vi "eyecat MAX v02_JS.vi"() -> ()   [LabVIEW 2014]
doc: "This VI is an upgrade from the WIN 1_v4 that implements the ageing subrutine"
uses:
  Buttons/String output.ctl
  <vilib>/Utility/miscctls.llb/LVRowAndColumnTypeDef.ctl
  Buttons/Numeric control.ctl
  Buttons/String input.ctl
  Buttons/Numeric indicator.ctl
  Controls Win/Control 3.ctl
  <vilib>/Platform/TimedLoop/XDataNode/nitl_modes.ctl
  <vilib>/Platform/TimedLoop/XDataNode/timing_clust.ctl
  <vilib>/Platform/TimedLoop/XDataNode/wakeup.ctl
  <vilib>/Utility/file.llb/Read From Spreadsheet File (DBL).vi
  <vilib>/Utility/file.llb/Write To Spreadsheet File (string).vi
  <vilib>/Utility/file.llb/Read From Spreadsheet File (string).vi
  <vilib>/regexp/Match Regular Expression.xnode
  <vilib>/Platform/TimedLoop/XDataNode/XDataNode.xnode
  <vilib>/Platform/TimedLoop/XDataNode/XDNodeRunTimeDep.lvlib
panel:
  out "SO Valve 2":dbl[][](array[numeric]) format="%0.3f"
  out "SO Valve 1":dbl[][](array[numeric]) format="%0.3f"
  out "File name":string
  out "Log?":bool
  out "Advanced Logging":bool
  out "output cluster":T2
  out "Connected":bool
  out "Air Bal Array":dbl[][](array[numeric]) format="%0.3f"
  out "HC Array Bal":dbl[][](array[numeric]) format="%0.3f"
  out "Air Array":dbl[][](array[numeric]) format="%0.3f"
  out "HC Array Cyc":dbl[][](array[numeric]) format="%0.3f"
  out "MKS 1":i16
  out "MKS 2":i16
  out "Furnace temp 2":dbl
  out "Full system?":bool
  out "Log interval (seconds)":T1
  in  "Flow rate Age":dbl
  in  "Inlet temp Age":dbl
  out "Stopped?":bool
  in  "Stop Cmd":T1
  out "Connected?":bool
  out "Error":dbl
  out "Iteration Duration":i64
  out "Finished Late? [i-1]":bool
  in  "stop TCP":bool
  in  "SO2 ppm":dbl
  out "Furnace temp 1":dbl
  out "stop 2":bool
  in  "Enum 1":i16=1
  in  "Acknowledge":bool
  out "Test number":u16
  out "Flag1":bool=TRUE
  out "EditPos Subc":T3
  out "Flag 2":bool=TRUE
  in  "Tab Control":T4(tab)
  out "Doors Unlocked":bool
  in  "Temperature Limit (°C)":T1=800.0 min=0.0 max=1200.0 step=1.0
  in  "Log Test Button":bool
  in  "File Name":T5="Test"
  in  "File Path":path=path "C:/DATA LOG"
  out "Fail":bool
  out "Pass":bool
  in  "Select Test Type":T6(radio)
  out "Standby":bool
  out "Doors Open":bool
  out "Extractor Fan On":bool
  out "Test In Progress":bool
  out "Cool Down":bool
  out "System Alarm":bool
  in  "Execute Leak Test Button":bool
  in  "Stop Test Button":bool
  in  "Start Test Button":bool
  in  "Advanced settings":bool
  in  "Inlet Temperature (°C)":T1=400.0 min=350.0 max=1000.0 step=1.0
  in  "Inlet LAMBDA Rich":T1=0.9 min=0.85 max=0.96 step=0.001
  in  "Inlet LAMBDA Lean":T1=1.2 min=1.02 max=3.0 step=0.001
  in  "Test Stop temperature (°C)":T1=300.0 min=100.0 max=1000.0 step=1.0
  in  "Test Start Temperature (°C)":T1=125.0 min=0.0 max=500.0 step=1.0
  in  "Furnace Ramp Rate (°C/min)":T1=15.0 min=1.0 max=50.0 step=0.1
  in  "NO:CO Ratio":T1=1.1 min=1.0 max=5.0 step=0.1
  in  "Inlet O2 (%)":T1=0.5 min=0.0 max=14.0 step=0.01
  in  "Inlet LAMBDA":T1=1.0 min=0.6 max=3.0 step=0.001
  out "Space Velocity (h-1)":T7
  out "Vol Flow @ STP (l/min)":T7
  in  "Test Flow Rate(g/s)":T1 min=0.0 max=100.0 step=0.01
  out "Sample Volume (litres)":T7
  in  "Number of Samples":T1=1.0 min=1.0 max=6.0 step=1.0
  in  "Sample Diameter (mm)":T1
  out "CO Theory (%)":T7 format="%#_3g"
  out "CO Theory (%)":T7 format="%#_3g"
  out "HC Theory (%)":T7
  in  "Sample Length (mm)":T1 min=0.0 step=0.5
  in  "NO ppm SW":dbl=500.0 caption="NO (ppm)" min=0.0 max=500.0 step=1.0
  in  "NO ppm Loff":T1 caption="NO ppm"
  in  "Delete sCycle":bool
  in  "Load sCycle":bool
  in  "Save sCycle":bool
  in  "Clear subcycle":bool
  in  "Clear Cycle Pattern":bool
  in  "Save Cycle":bool
  in  "Load Cycle":bool
  in  "Delete Cycle":bool
  out "Test Compiled":bool
  in  "Compile Test Button":bool
  in  "Sub-Cycle List":i32(listbox)=1
  in  "Cycle List":i32(listbox)=2
  out "Total Test Duration (hrs)":T8
  in  "Ageing Gas":enum32{"Radio Selection 1", "Radio Selection 2"}(radio)
  in  "Sub-Cycle Pattern":string[][](table) caption="Subcycle pattern"
  in  "Total Number of Cycles":T1=1.0 min=1.0 max=10000.0 step=1.0
  in  "Cycle Pattern":string[][](table)
  in  "Sub-Cycle Name":T5
  in  "Cycle Name":T5
  out "Heat Exchanger Temperatures (°C)":dynamicdata(graph)
  out "Flow Rate (g/s)":dynamicdata(graph)
  out "Sample Temperatures (°C)":dynamicdata(graph)
  out "System Temperatures (°C)":dynamicdata(graph)
  out "HC Concentration (ppm)":dynamicdata(graph)
  out "Lambda":dynamicdata(graph)
  out "M584L Upstream & Downstream":dynamicdata(graph)
  out "NO Concentration (ppm)":dynamicdata(graph)
  in  "Purge System":bool
  in  "Alarm ack":bool
  in  "Clear log":bool
  out "Table":string[][](table)
  out "Soft Alarm":bool
  out "Hard Alarm":bool
  # "Test Type"
  # "Test Commands"
  # "System Indicators"
  # "Leak Test"
  # "Catalyst Specification"
  # "Lightoff Settings"
  # "Furnace Lightoff Settings"
  # "Sweep Settings"
  # "CO/HC Lightoff Settings"
  # "0.96 < lambda < 0.85"
  # "1.02< lambda < 1.6"
  # "350 < Tinlet < 1000"
  # "NO Lightoff Settings"
  # "Flow Specification"
  # "Cycle Compiled"
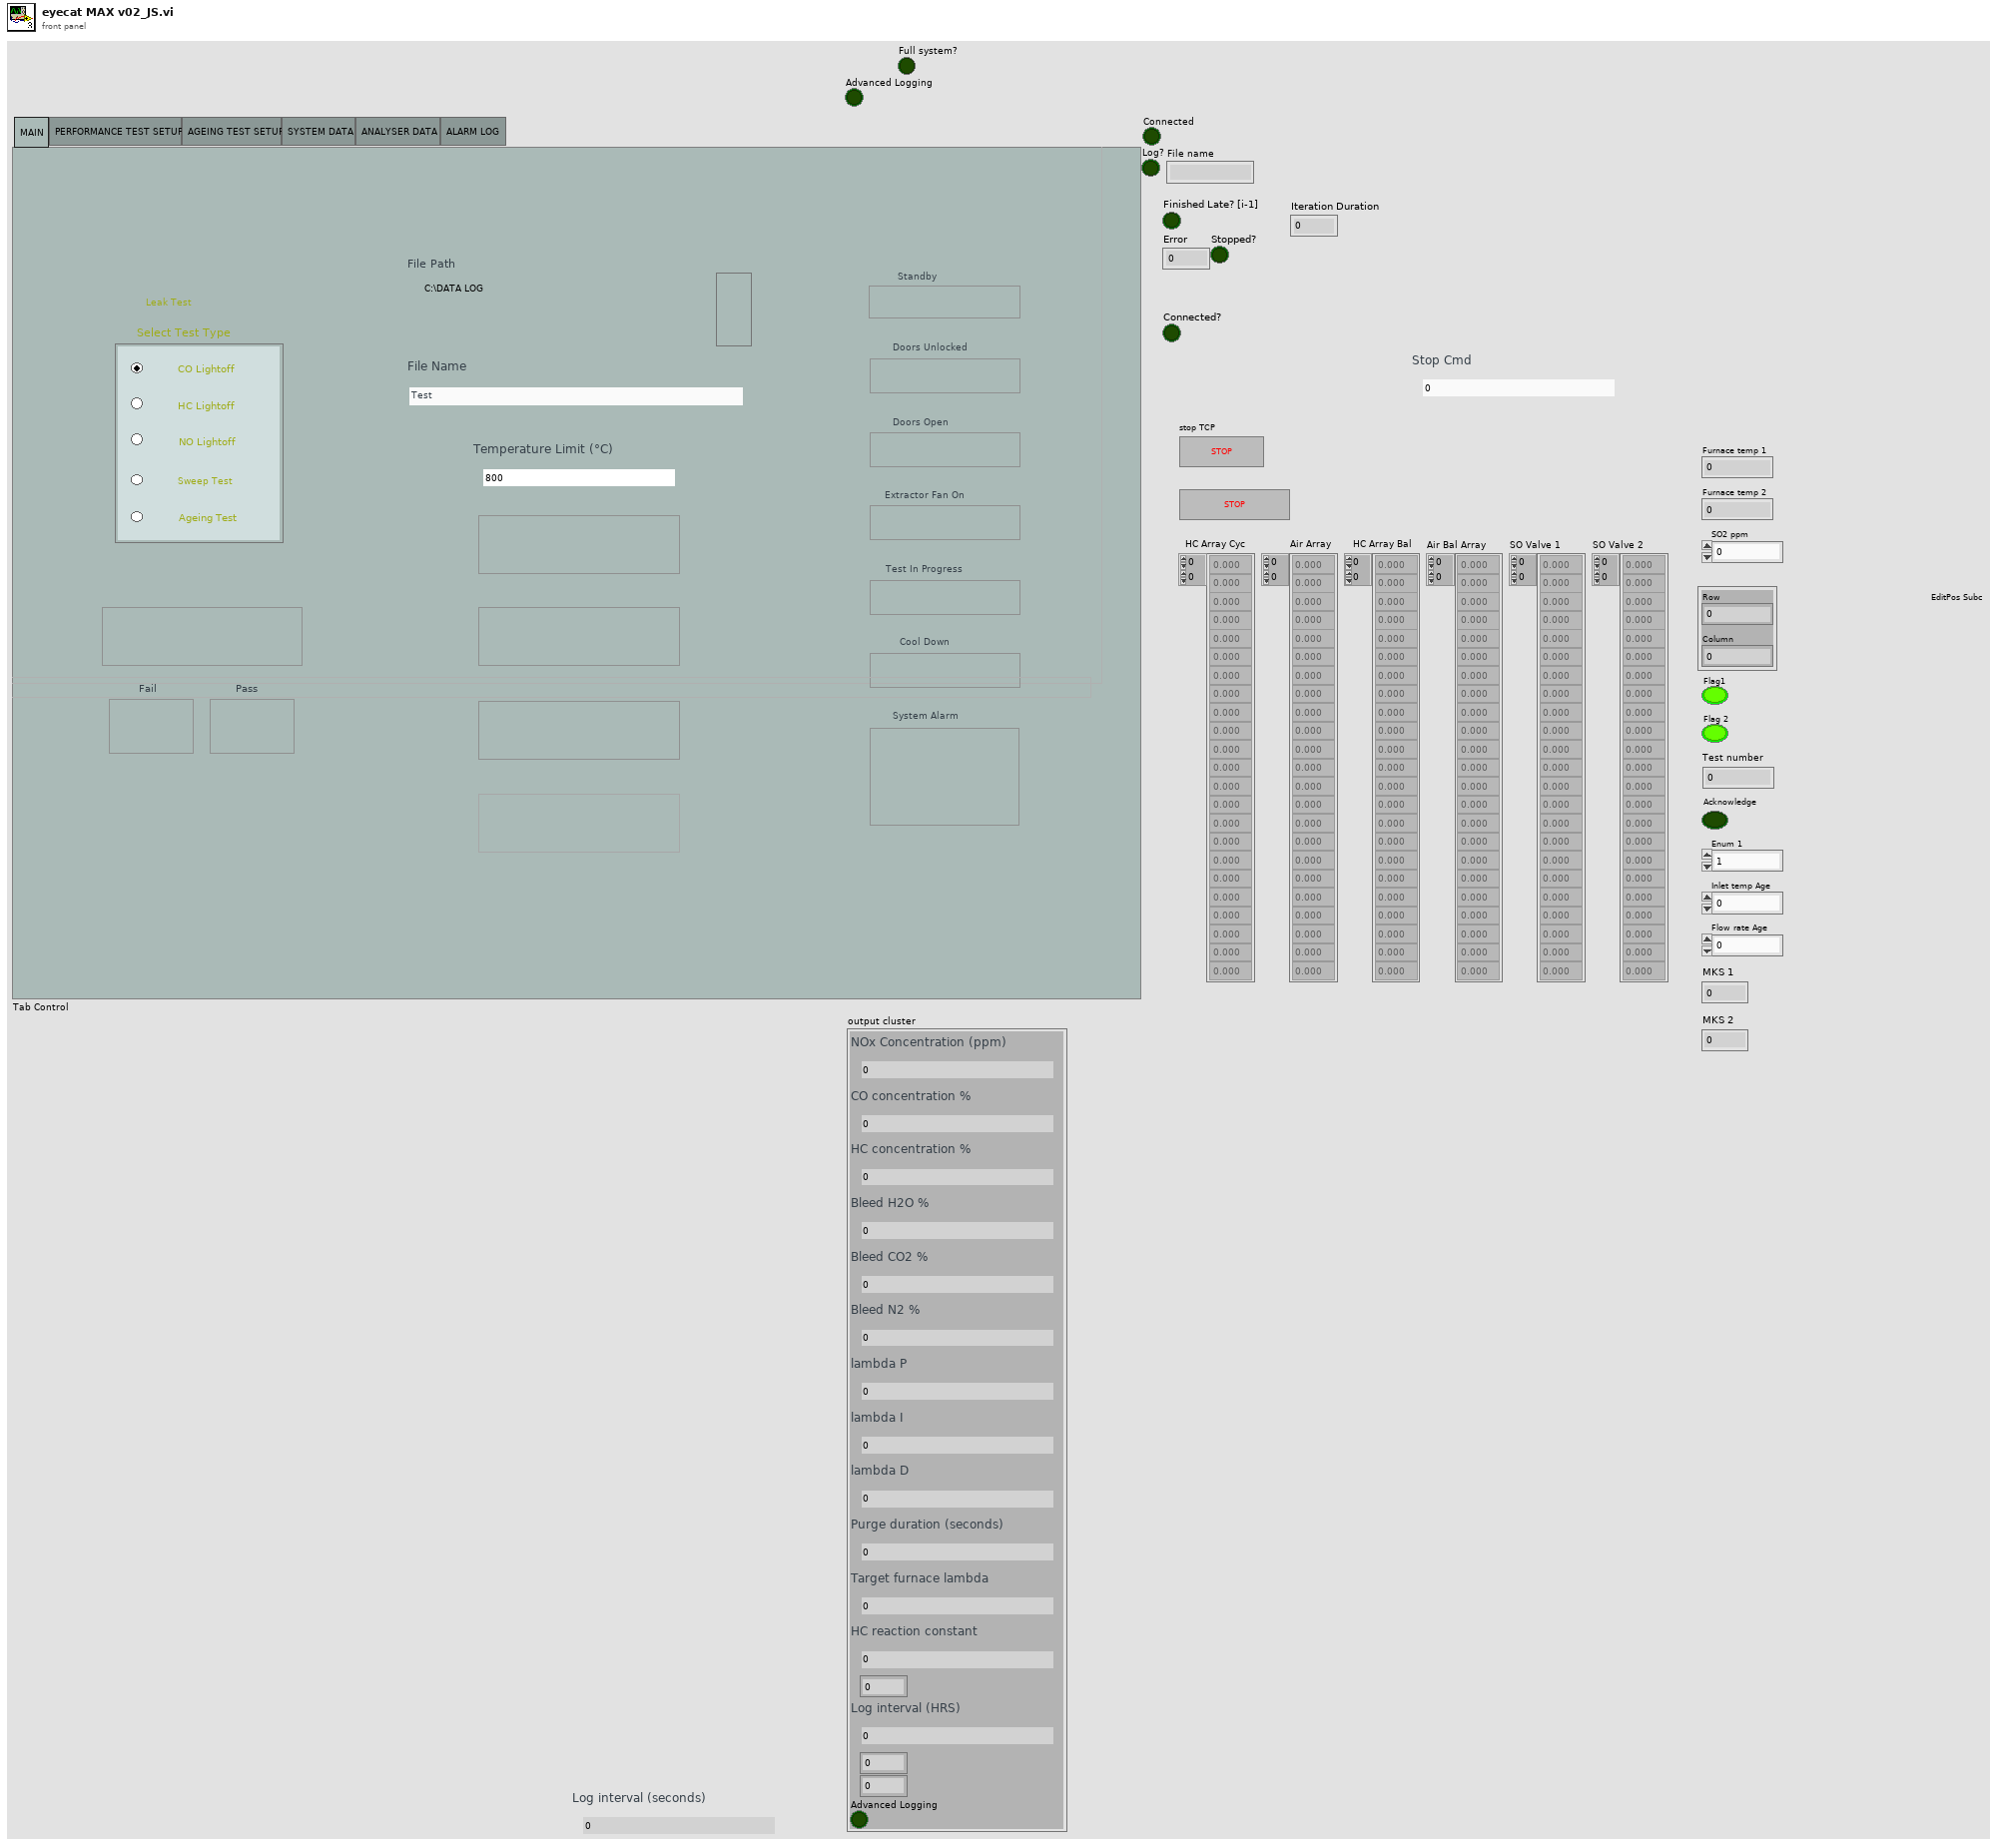
[diagram p1: front panel]
types:
  T1 = typedef "Numeric control.ctl" = dbl
  T2 = cluster{"NOx Concentration (ppm)":T1, "CO concentration %":T1, "HC concentration %":T1, "Bleed H2O %":T1, "Bleed CO2 %":T1, "Bleed N2 %":T1, "lambda P":T1, "lambda I":T1, "lambda D":T1, "Purge duration (seconds)":T1, "Target furnace lambda":T1, "HC reaction constant":T1, i16, "Log interval (HRS)":T1, i16, i16, "Advanced Logging":bool}
  T3 = typedef "LVRowAndColumnTypeDef.ctl" = cluster{"Row":i32, "Column":i32}
  T4 = enum32{"MAIN", "PERFORMANCE TEST SETUP", "AGEING TEST SETUP", "SYSTEM DATA", "ANALYSER DATA", "ALARM LOG"}
  T5 = typedef "String input.ctl" = string
  T6 = enum32{"CO Lightoff", "HC Lightoff", "NO Lightoff", "Sweep Test", "Ageing Test"}
  T7 = typedef "Numeric indicator.ctl" = dbl
  T8 = typedef "String output.ctl" = string
  T9 = typedef "XDNodeRunTimeDep.lvlib/nitl_modes.ctl" = enum32{"No Change", "Process missed periods, maintain original phase", "Discard missed periods, maintain original phase", "Process missed periods, ignore original phase", "Discard missed periods, ignore original phase"}
  T10 = typedef "Control 3.ctl" = enum16{"main", "start test", "save subc", "load subc", "delete subc", "clear table 1", "update list 1", "save cycle", "load cycle", "delete cycle", "clear table 2", "update list 2", "calc HC CO", "Total time calc", "update Cycle pattern ", "load cycle name", "convert to num", "load test array", "check scycle name", "check cycle name", "Multigas connect", "Multigas disconnect"}
  T11 = enum8{"Enabled", "Disabled", "Disabled and Grayed Out"}
  T12 = typedef "XDNodeRunTimeDep.lvlib/timing_clust.ctl" = cluster{"Expected End [f-1]":u64, "Actual End [f-1]":u64, "Finished Late? [f-1]":bool, "Expected End [i-1]":u64, "Actual End [i-1]":u64, "Finished Late? [i-1]":bool, "Expected Start [i]":u64, "Actual Start [i]":u64, "Expected Start [f]":u64, "Actual Start [f]":u64, "Source Name":string, "Structure Name":string, "Period":i64, "Deadline":i64, "Offset":i64, "Start":i64, "Priority":i32, "Timeout":i32, "Mode":T9, "Wakeup Reason":T13, "Error":errorcluster, "Source Type":string, "Secondary Source Type":string, "Global End Time":u64, "Global Start Time":u64, "Frame Duration":u64, "Iteration Duration":u64, "Assigned CPU":i32, "I/O Scan Engine Mode":u32}
  T13 = typedef "XDNodeRunTimeDep.lvlib/wakeup.ctl" = enum32{"Normal", "Aborted", "Asynchronous wakeup", "Timing source error", "Timed loop error", "Timeout"}
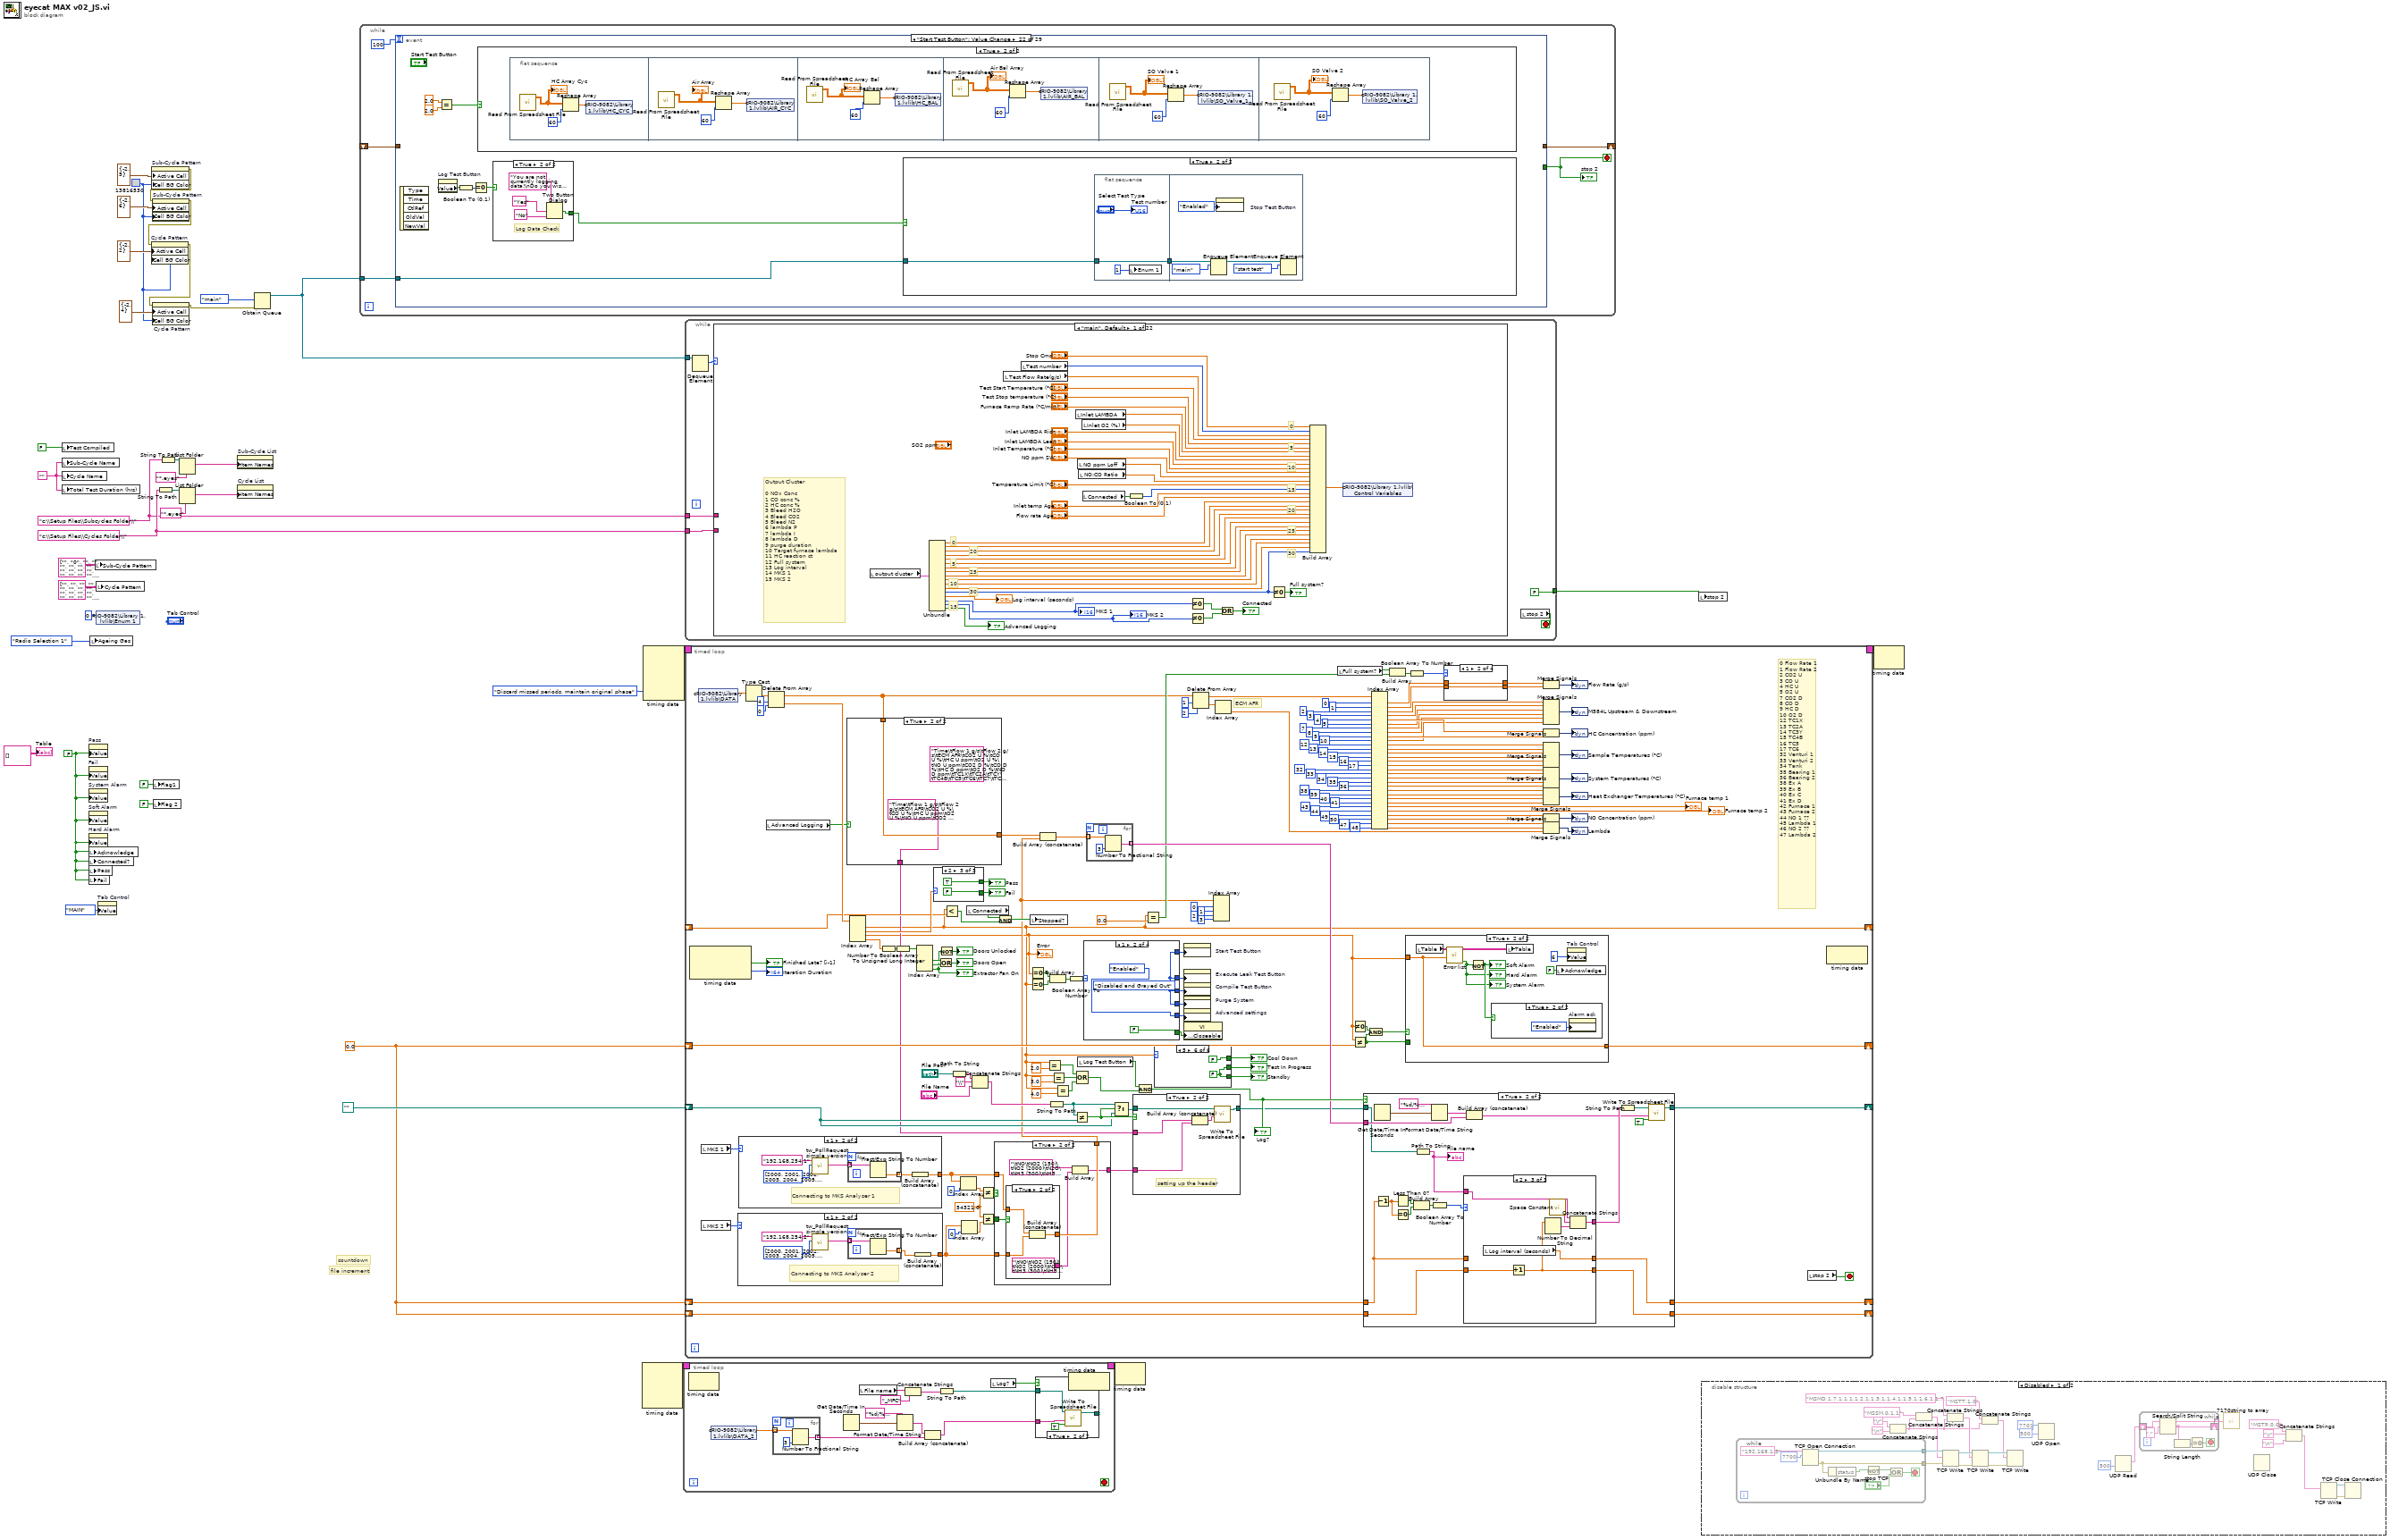
[diagram p0: block diagram]
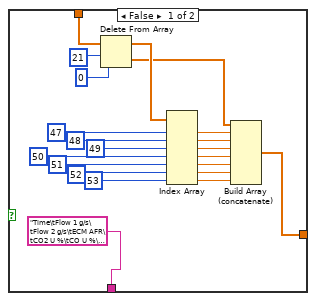
[diagram p4: hidden frame]
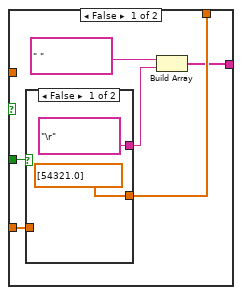
[diagram p5: hidden frame]
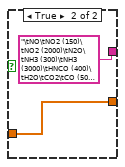
[diagram p6: hidden frame]
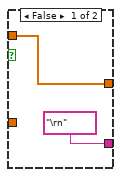
[diagram p7: hidden frame]
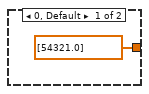
[diagram p8: hidden frame]
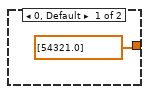
[diagram p9: hidden frame]
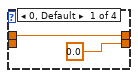
[diagram p10: hidden frame]
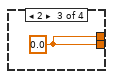
[diagram p11: hidden frame]
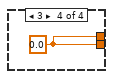
[diagram p12: hidden frame]
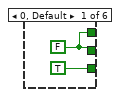
[diagram p13: hidden frame]
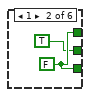
[diagram p14: hidden frame]
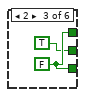
[diagram p15: hidden frame]
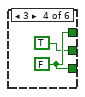
[diagram p16: hidden frame]
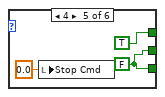
[diagram p17: hidden frame]
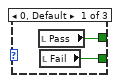
[diagram p18: hidden frame]
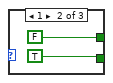
[diagram p19: hidden frame]
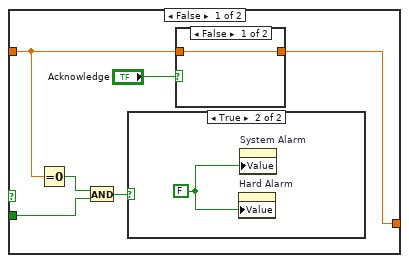
[diagram p20: hidden frame]
diagram:
  w4 = FALSE
  w3 = 0.0 ("y")
  w20 = ""
  w23 = "c:\\Setup Files\\Cycles Folder\\"
  w29 = u32 13816530
  w21 = "c:\\Setup Files\\Subcycles Folder\\"
  # "file increment"
  # "countdown"
  n1 = local write "Test Compiled"(FALSE ("Cycle Compiled")) -> ()
  n2 = local write "Sub-Cycle Name"(w20) -> ()
  n3 = local write "Cycle Name"(w20) -> ()
  n4 = local write "Total Test Duration (hrs)"(w20) -> ()
  n5 = property on="Pass" class="Bool (strict)"("Value"=w4) -> ()  [unwired: 2 in, 2 out]
  n6 = property on="Fail" class="Bool (strict)"("Value"=w4) -> ()  [unwired: 2 in, 2 out]
  n7 = property on="System Alarm" class="Bool (strict)"("Value"=w4) -> ()  [unwired: 2 in, 2 out]
  n8 = property on="Soft Alarm" class="Bool (strict)"("Value"=w4) -> ()  [unwired: 2 in, 2 out]
  n9 = property on="Hard Alarm" class="Bool (strict)"("Value"=w4) -> ()  [unwired: 2 in, 2 out]
  n10 = local write "Acknowledge"(w4) -> ()
  n11 = local write "Connected?"(w4) -> ()
  n12 = local write "Pass"(w4) -> ()
  n13 = local write "Fail"(w4) -> ()
  n14 = local write "Ageing Gas"(enum32{"Radio Selection 1", "Radio Selection 2"}."Radio Selection 1" ("Ageing Gas")) -> ()
  n15 = local write "Sub-Cycle Pattern"(string[][] [["", "0", "", "", "", "", "", "", "", "", "", "", ""], ["", "", "", "", "", "", "", "", "", "", "", "", ""], ["", "", "", "", "", "", "", "", "", "", "", "", ""], ["", "", "", "", "", "", "", "", "", "", "", "", ""], ["", "", "", "", "", "", "", "", "", "", "", "", ""], ["", "", "", "", "", "", "", "", "", "", "", "", ""], ["", "", "", "", "", "", "", "", "", "", "", "", ""], ["", "", "", "", "", "", "", "", "", "", "", "", ""], ["", "", "", "", "", "", "", "", "", "", "", "", ""], ["", "", "", "", "", "", "", "", "", "", "", "", ""], ["", "", "", "", "", "", "", "", "", "", "", "", ""], ["", "", "", "", "", "", "", "", "", "", "", "", ""], ["", "", "", "", "", "", "", "", "", "", "", "", ""], ["", "", "", "", "", "", "", "", "", "", "", "", ""], ["", "", "", "", "", "", "", "", "", "", "", "", ""], ["", "", "", "", "", "", "", "", "", "", "", "", ""], ["", "", "", "", "", "", "", "", "", "", "", "", ""], ["", "", "", "", "", "", "", "", "", "", "", "", ""], ["", "", "", "", "", "", "", "", "", "", "", "", ""], ["", "", "", "", "", "", "", "", "", "", "", "", ""], ["", "", "", "", "", "", "", "", "", "", "", "", ""], ["", "", "", "", "", "", "", "", "", "", "", "", ""], ["", "", "", "", "", "", "", "", "", "", "", "", ""], ["", "", "", "", "", "", "", "", "", "", "", "", ""], ["", "", "", "", "", "", "", "", "", "", "", "", ""], ["", "", "", "", "", "", "", "", "", "", "", "", ""], ["", "", "", "", "", "", "", "", "", "", "", "", ""], ["", "", "", "", "", "", "", "", "", "", "", "", ""], ["", "", "", "", "", "", "", "", "", "", "", "", ""], ["", "", "", "", "", "", "", "", "", "", "", "", ""], ["", "", "", "", "", "", "", "", "", "", "", "", ""]]) -> ()
  n16 = local write "Cycle Pattern"(string[][] [["", "", "", "", ""], ["", "", "", "", ""], ["", "", "", "", ""], ["", "", "", "", ""], ["", "", "", "", ""], ["", "", "", "", ""], ["", "", "", "", ""], ["", "", "", "", ""], ["", "", "", "", ""], ["", "", "", "", ""], ["", "", "", "", ""], ["", "", "", "", ""], ["", "", "", "", ""], ["", "", "", "", ""], ["", "", "", "", ""], ["", "", "", "", ""], ["", "", "", "", ""], ["", "", "", "", ""], ["", "", "", "", ""], ["", "", "", "", ""], ["", "", "", "", ""], ["", "", "", "", ""], ["", "", "", "", ""], ["", "", "", "", ""], ["", "", "", "", ""], ["", "", "", "", ""], ["", "", "", "", ""], ["", "", "", "", ""], ["", "", "", "", ""], ["", "", "", "", ""], ["", "", "", "", ""]]) -> ()
  n17 = shared-variable "cRIO-9082\\Library 1.lvlib\\Enum 1"(u16 0 ("Enum 1")) -> ()  [unwired: 1 in, 1 out]
  n18 = property on="Tab Control" class="TabCtl (strict)"("Value"=T4."MAIN" ("Tab Control")) -> ()  [unwired: 2 in, 2 out]
  n19 = property on="Sub-Cycle Pattern" class="Tbl (strict)"("Active Cell"=T3 {"Row"=-2, "Column"=5} ("Active Cell:Active Cell"), "Cell BG Color"=w29) -> (error out=w34:errorcluster)  [unwired: 2 in, 1 out]
  n20 = property on="Sub-Cycle Pattern" class="Tbl (strict)"(error in=w34, "Active Cell"=T3 {"Row"=-2, "Column"=6} ("Active Cell:Active Cell"), "Cell BG Color"=w29) -> (error out=w33:errorcluster)  [unwired: 1 in, 1 out]
  n21 = property on="Cycle Pattern" class="Tbl (strict)"(error in=w33, "Active Cell"=T3 {"Row"=-2, "Column"=2} ("Active Cell:Active Cell"), "Cell BG Color"=w29) -> (error out=w31:errorcluster)  [unwired: 1 in, 1 out]
  n22 = property on="Cycle Pattern" class="Tbl (strict)"(error in=w31, "Active Cell"=T3 {"Row"=-2, "Column"=4} ("Active Cell:Active Cell"), "Cell BG Color"=w29) -> (error out=w28:errorcluster)  [unwired: 1 in, 1 out]
  n23 = local write "Flag1"(FALSE) -> ()
  n24 = local write "Flag 2"(FALSE) -> ()
  n25 = String To Path(string=w23) -> (path=w24:path)
  n26 = String To Path(string=w21) -> (path=w26:path)
  n27 = List Folder(path=w24, pattern="*.eyec") -> (filenames=w25:string[])  [unwired: 2 in, 3 out]
  n28 = List Folder(path=w26, pattern="*.eyes") -> (filenames=w27:string[])  [unwired: 2 in, 3 out]
  n29 = property on="Sub-Cycle List" class="LstBox (strict)"("Item Names"=w27) -> ()  [unwired: 2 in, 2 out]
  n30 = property on="Cycle List" class="LstBox (strict)"("Item Names"=w25) -> ()  [unwired: 2 in, 2 out]
  n31 = Obtain Queue(element data type=Control_3."main" ("Enum"), error in (no error)=w28) -> (queue out=w37:refnum<queue>)  [unwired: 3 in, 2 out]
  n32 = while {
    tunnel: w37 -> [w43]
    shift-right: [w41] -> _
    shift-left: _ -> [w40]
    stop <- w39 stop-if-true
    n33 = event shown="[21] \"Start Test Button\": Value Change" {
      selector: _ -> [_ _ _ _ _ _ _ _ _ _ _ _ _ _ _ _ _ _ _ _ _ _ _ _ _ _ _ _ _]
      dyn-events: _ -> [_ _ _ _ _ _ _ _ _ _ _ _ _ _ _ _ _ _ _ _ _ _ _ _ _ _ _ _ _]
      timeout: 100 -> [_ _ _ _ _ _ _ _ _ _ _ _ _ _ _ _ _ _ _ _ _ _ _ _ _ _ _ _ _]
      tunnel: w43 -> [w46 w48 _ w57 w65 w72 w79 w90 w94 w105 w110 w113 w118 w140 w148 w149 _ _ _ _ w193 w208 _ w251 w269 _ w283 _ _]
      tunnel: [w44 w47 _ w58 w64 w71 w78 w89 w92 w100 w107 w112 w116 w137 _ _ _ _ _ _ _ _ _ _ _ _ _ _ _] -> w41
      tunnel: w40 -> [w44 w47 _ w58 w64 w71 w77 w89 w92 w100 w107 w112 w116 w137 _ _ _ _ _ _ _ _ _ _ _ _ _ _ _]
      tunnel: [_ _ w50 _ _ _ _ _ _ _ _ _ _ _ _ _ _ _ _ _ _ _ _ _ _ _ _ _ _] -> w39
      event Timeout {
        n34 = event-data() -> ()  [unwired: 1 in, 2 out]
        n35 = Enqueue Element(queue=w46, element=Control_3."main" ("Enum")) -> ()  [unwired: 2 in, 3 out]
      }
      event "Clear subcycle": Value Change {
        n36 = event-data() -> ()  [unwired: 1 in, 5 out]
        n37 = Enqueue Element(queue=w48, element=Control_3."clear table 1" ("Enum")) -> ()  [unwired: 2 in, 3 out]
      }
      event Panel Close? {
        n38 = event-data() -> ()  [unwired: 1 in, 3 out]
        n39 = Two Button Dialog(message="This command will close Eyecat!\nDo you wish to continue?", 1:"No" ("F button name (\"Cancel\")"), 2:"Yes" ("T button name (\"OK\")")) -> (T button?=w50:bool)
        n40 = Not(x=w50) -> (.not. x?=w51:bool)
        n41 = event-data("Discard?"=w51) -> ()  [unwired: 1 in, 1 out]
      }
      event "Save sCycle": Value Change {
        n42 = event-data() -> ()  [unwired: 1 in, 5 out]
        n43 = local read "Sub-Cycle Pattern"() -> (w55:string[][])
        n44 = call "Time column check.vi"("Array"=w55) -> ("Mistake?"=w56:bool)  [unwired: 10 in]
        n45 = case shown="False" w56 {
          tunnel: w57 -> [w59 _]
          frame False {
            n46 = Enqueue Element(queue=w59, element=Control_3."save subc") -> (queue out=w61:refnum<queue>)  [unwired: 2 in, 2 out]
            n47 = Enqueue Element(queue=w61, element=Control_3."update list 1") -> ()  [unwired: 2 in, 3 out]
          }
          frame True {
            n48 = One Button Dialog(message="The time sequence is incorrect!\nReview and save again!") -> ()  [unwired: 1 in, 1 out]
          }
        }
      }
      event "Load sCycle": Value Change {
        n49 = event-data() -> ()  [unwired: 1 in, 5 out]
        n50 = Enqueue Element(queue=w65, element=Control_3."load subc") -> ()  [unwired: 2 in, 3 out]
      }
      event "Delete sCycle": Value Change {
        n51 = event-data() -> ()  [unwired: 1 in, 5 out]
        n52 = Enqueue Element(queue=w72, element=Control_3."delete subc") -> (queue out=w74:refnum<queue>)  [unwired: 2 in, 2 out]
        n53 = Enqueue Element(queue=w74, element=Control_3."update list 1") -> (queue out=w70:refnum<queue>)  [unwired: 2 in, 2 out]
        n54 = Enqueue Element(queue=w70, element=Control_3."update Cycle pattern ") -> (queue out=w67:refnum<queue>)  [unwired: 2 in, 2 out]
        n55 = Enqueue Element(queue=w67, element=Control_3."Total time calc") -> ()  [unwired: 2 in, 3 out]
      }
      event "Sub-Cycle Pattern": Mouse Down; "Sub-Cycle Pattern": Value Change {
        n56 = event-data() -> ()  [unwired: 1 in, 3 out]
        n57 = property on="Sub-Cycle Pattern" class="Tbl (strict)"() -> ("EditPos"=w78:T3)  [unwired: 2 in, 2 out]
        n58 = Unbundle By Name(w78) -> ("Row"=w80:i32)  [unwired: 1 out]
        n59 = Less?(x=w80, y=30) -> (x < y?=w82:bool)
        n60 = case shown="True" w82 {
          tunnel: w79 -> [_ w87]
          frame False {
            n61 = One Button Dialog(message="This table is limited to 30 entries!") -> ()  [unwired: 1 in, 1 out]
          }
          frame True {
            n62 = Enqueue Element(queue=w87, element=Control_3."convert to num") -> (queue out=w86:refnum<queue>)  [unwired: 2 in, 2 out]
            n63 = Enqueue Element(queue=w86, element=Control_3."calc HC CO") -> ()  [unwired: 2 in, 3 out]
          }
        }
        "EditPos Subc" <- w77
        "Flag1" <- TRUE
      }
      event "Clear Cycle Pattern": Value Change {
        n64 = event-data() -> ()  [unwired: 1 in, 5 out]
        n65 = Enqueue Element(queue=w90, element=Control_3."clear table 2" ("Enum")) -> ()  [unwired: 2 in, 3 out]
        n66 = local write "Test Compiled"(FALSE ("Test Compiled")) -> ()
      }
      event "Save Cycle": Value Change {
        n67 = event-data() -> ()  [unwired: 1 in, 5 out]
        n68 = Enqueue Element(queue=w94, element=Control_3."update Cycle pattern ") -> (queue out=w93:refnum<queue>)  [unwired: 2 in, 2 out]
        n69 = Enqueue Element(queue=w93, element=Control_3."save cycle") -> (queue out=w97:refnum<queue>)  [unwired: 2 in, 2 out]
        n70 = Enqueue Element(queue=w97, element=Control_3."update list 2") -> ()  [unwired: 2 in, 3 out]
      }
      event "Load Cycle": Value Change {
        n71 = event-data() -> ()  [unwired: 1 in, 5 out]
        n72 = Enqueue Element(queue=w105, element=Control_3."load cycle") -> (queue out=w103:refnum<queue>)  [unwired: 2 in, 2 out]
        n73 = Enqueue Element(queue=w103, element=Control_3."update Cycle pattern ") -> (queue out=w102:refnum<queue>)  [unwired: 2 in, 2 out]
        n74 = local write "Test Compiled"(FALSE ("Test Compiled")) -> ()
        n75 = Enqueue Element(queue=w102, element=Control_3."Total time calc") -> ()  [unwired: 2 in, 3 out]
      }
      event "Delete Cycle": Value Change {
        n76 = event-data() -> ()  [unwired: 1 in, 5 out]
        n77 = Enqueue Element(queue=w110, element=Control_3."delete cycle") -> (queue out=w109:refnum<queue>)  [unwired: 2 in, 2 out]
        n78 = Enqueue Element(queue=w109, element=Control_3."update list 2") -> ()  [unwired: 2 in, 3 out]
      }
      event Value Change {
        n79 = event-data() -> ()  [unwired: 1 in, 5 out]
        n80 = Enqueue Element(queue=w113, element=Control_3."Total time calc") -> ()  [unwired: 2 in, 3 out]
      }
      event "Cycle Pattern": Mouse Up; "Cycle Pattern": Value Change {
        n81 = event-data() -> ()  [unwired: 1 in, 3 out]
        n82 = property on="Cycle Pattern" class="Tbl (strict)"() -> ("EditPos"=w120:T3)  [unwired: 2 in, 2 out]
        n83 = Unbundle By Name(w120) -> ("Row"=w117:i32, "Column"=w122:i32)
        n84 = Less?(x=w117, y=30) -> (x < y?=w121:bool)
        n85 = case shown="True" w121 {
          tunnel: w122 -> [_ w124]
          tunnel: w118 -> [_ w127]
          frame False {
            n86 = One Button Dialog(message="This table is limited to 30 entries!") -> ()  [unwired: 1 in, 1 out]
          }
          frame True {
            n87 = Equal?(x=w124, y=1) -> (x = y?=w128:bool)
            n88 = case shown="True" w128 {
              tunnel: w127 -> [w131 w134]
              tunnel: [w130 w133] -> w126
              frame False {
                n89 = Enqueue Element(queue=w131, element=Control_3."update Cycle pattern ") -> (queue out=w130:refnum<queue>)  [unwired: 2 in, 2 out]
              }
              frame True {
                n90 = Enqueue Element(queue=w134, element=Control_3."load cycle name") -> (queue out=w133:refnum<queue>)  [unwired: 2 in, 2 out]
              }
            }
            n91 = Enqueue Element(queue=w126, element=Control_3."Total time calc") -> ()  [unwired: 2 in, 3 out]
          }
        }
        "Flag 2" <- TRUE
      }
      event "Compile Test Button": Value Change {
        n92 = event-data() -> ()  [unwired: 1 in, 5 out]
        n93 = local read "Flag 2"() -> (w136:bool)
        n94 = case shown="True" w136 {
          tunnel: w140 -> [w141 w145]
          tunnel: [w141 w142] -> w138
          frame False {
          }
          frame True {
            n95 = Enqueue Element(queue=w145, element=Control_3."save cycle") -> (queue out=w143:refnum<queue>)  [unwired: 2 in, 2 out]
            n96 = Enqueue Element(queue=w143, element=Control_3."update list 2") -> (queue out=w142:refnum<queue>)  [unwired: 2 in, 2 out]
          }
        }
        n97 = Enqueue Element(queue=w138, element=Control_3."load test array") -> ()  [unwired: 2 in, 3 out]
      }
      event Value Change {
        n98 = event-data() -> ()  [unwired: 1 in, 5 out]
        n99 = Enqueue Element(queue=w148, element=Control_3."check scycle name") -> ()  [unwired: 2 in, 3 out]
      }
      event Value Change {
        n100 = event-data() -> ()  [unwired: 1 in, 5 out]
        n101 = Enqueue Element(queue=w149, element=Control_3."check cycle name") -> ()  [unwired: 2 in, 3 out]
      }
      event Value Change {
        n102 = event-data() -> ()  [unwired: 1 in, 5 out]
        n103 = Square(x="Sample Diameter (mm)") -> (x^2=w158:T1)
        n104 = Compound Arithmetic op=MULTIPLY(w158, "Sample Length (mm)", "Number of Samples", 3.141592653589793) -> (w157:T1)
        n105 = Divide(x=w157, y=4000000.0) -> (x/y=→"Sample Volume (litres)":T1)
      }
      event Value Change {
        # "O2Eq"
        n106 = event-data() -> ()  [unwired: 1 in, 5 out]
        n107 = local write "Inlet LAMBDA"("Inlet LAMBDA") -> ()
        n108 = local write "Inlet O2 (%)"("Inlet O2 (%)") -> ()
        n109 = Decrement(x="Inlet LAMBDA") -> (x-1=w173:T1)
        n110 = Multiply(x=4.76, y="Inlet LAMBDA") -> (x*y=w169:T1)
        n111 = Multiply(x=w173, y=100.0) -> (x*y=w171:T1)
        n112 = Add(x=0.33, y=w169) -> (x+y=w167:T1)
        n113 = Divide(x=w171, y=w167) -> (x/y=w166:T1)
        n114 = Subtract(x="Inlet O2 (%)", y=w166) -> (x-y=w164:T1)
        n115 = Multiply(x=w164, y=2.0) -> (x*y=→"CO Theory (%)":T1)
        n116 = Divide(x=w164, y=4.5) -> (x/y=→"HC Theory (%)":T1)
      }
      event Value Change {
        n117 = event-data() -> ()  [unwired: 1 in, 5 out]
        n118 = local write "NO ppm Loff"("NO ppm Loff") -> ()
        n119 = local write "NO:CO Ratio"("NO:CO Ratio") -> ()
        n120 = Divide(x="NO ppm Loff", y=T1 10000.0) -> (x/y=w176:T1)
        n121 = Multiply(x="NO:CO Ratio", y=w176) -> (x*y=→"CO Theory (%)":T1)
      }
      event Value Change {
        n122 = event-data() -> ()  [unwired: 1 in, 5 out]
        n123 = local read "Sample Volume (litres)"() -> (w181:T7)
        n124 = Equal?(x=w181, y=0.0) -> (x = y?=w180:bool)
        n125 = case shown="False" w180 {
          tunnel: w181 -> [w186 _]
          tunnel: "Test Flow Rate(g/s)" -> [w183 _]
          frame False {
            w188 = 60.0 ("y")
            n126 = Multiply(x=w183, y=w188) -> (x*y=w190:T1)
            n127 = Divide(x=w190, y=1.2) -> (x/y=w185:T1)
            "Vol Flow @ STP (l/min)" <- w185
            n128 = Multiply(x=w185, y=w188) -> (x*y=w187:T1)
            n129 = Divide(x=w187, y=w186) -> (x/y=→"Space Velocity (h-1)":T1)
          }
          frame True {
            n130 = One Button Dialog(message="Review sample specification first!") -> ()  [unwired: 1 in, 1 out]
          }
        }
      }
      event "Execute Leak Test Button": Value Change {
        n131 = event-data() -> ()  [unwired: 1 in, 5 out]
        n132 = flat-sequence {
          tunnel: w193 -> [w196]
          tunnel: [w196] -> w192
          tunnel: w192 -> [w199]
          frame #0 {
            n133 = local write "Test number"(u16 5) -> ()
            n134 = local write "Enum 1"(u16 3 ("Test number")) -> ()
          }
          frame #1 {
            n135 = Enqueue Element(queue=w199, element=Control_3."main" ("Enum")) -> (queue out=w197:refnum<queue>)  [unwired: 2 in, 2 out]
            n136 = Enqueue Element(queue=w197, element=Control_3."start test" ("Enum")) -> ()  [unwired: 2 in, 3 out]
          }
        }
      }
      event "Start Test Button": Value Change {
        n137 = event-data() -> ()  [unwired: 1 in, 5 out]
        n138 = property on="Log Test Button" class="Bool (strict)"() -> ("Value"=w207:bool)  [unwired: 2 in, 2 out]
        n139 = Equal?(x=2.0, y=2.0) -> (x = y?=w203:bool)
        n140 = Boolean To (0,1)(Boolean=w207) -> (0, 1=w206:i16)
        n141 = Equal To 0?(x=w206) -> (x = 0?=w205:bool)
        n142 = case shown="True" w203 {
          frame False {
          }
          frame True {
            n143 = flat-sequence {
              frame #0 {
                n144 = call-poly <vilib>:"Read From Spreadsheet File.vi"() -> ("all rows"=w211:dbl[][])  [unwired: 7 in, 4 out]
                "HC Array Cyc" <- w211
                n145 = Reshape Array(w211, 60 ("dimension size")) -> (w210:dbl[])
                n146 = shared-variable "cRIO-9082\\Library 1.lvlib\\HC_CYC"(w210) -> ()  [unwired: 1 in, 1 out]
              }
              frame #1 {
                n147 = call-poly <vilib>:"Read From Spreadsheet File.vi"() -> ("all rows"=w212:dbl[][])  [unwired: 7 in, 4 out]
                "Air Array" <- w212
                n148 = Reshape Array(w212, 60 ("dimension size")) -> (w214:dbl[])
                n149 = shared-variable "cRIO-9082\\Library 1.lvlib\\AIR_CYC"(w214) -> ()  [unwired: 1 in, 1 out]
              }
              frame #2 {
                n150 = call-poly <vilib>:"Read From Spreadsheet File.vi"() -> ("all rows"=w217:dbl[][])  [unwired: 7 in, 4 out]
                "HC Array Bal" <- w217
                n151 = Reshape Array(w217, 60 ("dimension size")) -> (w216:dbl[])
                n152 = shared-variable "cRIO-9082\\Library 1.lvlib\\HC_BAL"(w216) -> ()  [unwired: 1 in, 1 out]
              }
              frame #3 {
                n153 = call-poly <vilib>:"Read From Spreadsheet File.vi"() -> ("all rows"=w218:dbl[][])  [unwired: 7 in, 4 out]
                "Air Bal Array" <- w218
                n154 = Reshape Array(w218, 60 ("dimension size")) -> (w219:dbl[])
                n155 = shared-variable "cRIO-9082\\Library 1.lvlib\\AIR_BAL"(w219) -> ()  [unwired: 1 in, 1 out]
              }
              frame #4 {
                n156 = call-poly <vilib>:"Read From Spreadsheet File.vi"() -> ("all rows"=w223:dbl[][])  [unwired: 7 in, 4 out]
                "SO Valve 1" <- w223
                n157 = Reshape Array(w223, 60 ("dimension size")) -> (w222:dbl[])
                n158 = shared-variable "cRIO-9082\\Library 1.lvlib\\SO_Valve_1"(w222) -> ()  [unwired: 1 in, 1 out]
              }
              frame #5 {
                n159 = call-poly <vilib>:"Read From Spreadsheet File.vi"() -> ("all rows"=w224:dbl[][])  [unwired: 7 in, 4 out]
                "SO Valve 2" <- w224
                n160 = Reshape Array(w224, 60 ("dimension size")) -> (w225:dbl[])
                n161 = shared-variable "cRIO-9082\\Library 1.lvlib\\SO_Valve_2"(w225) -> ()  [unwired: 1 in, 1 out]
              }
            }
          }
        }
        n162 = case shown="True" w205 {
          tunnel: [TRUE ("T button?") w228] -> w204
          frame False {
          }
          frame True {
            # "Log Data Check"
            n163 = Two Button Dialog(message="You are not currently logging data!\nDo you wish to continue?", 1:"No" ("T button name (\"OK\")"), 2:"Yes" ("T button name (\"OK\")")) -> (T button?=w228:bool)
          }
        }
        n164 = case shown="True" w204 {
          tunnel: w208 -> [_ w233]
          frame False {
          }
          frame True {
            n165 = flat-sequence {
              tunnel: w233 -> [w236]
              tunnel: [w236] -> w232
              tunnel: w232 -> [w240]
              frame #0 {
                n166 = local write "Enum 1"(u16 1 ("Test number")) -> ()
                "Test number" <- "Select Test Type"
              }
              frame #1 {
                n167 = Enqueue Element(queue=w240, element=Control_3."main" ("Enum")) -> (queue out=w238:refnum<queue>)  [unwired: 2 in, 2 out]
                n168 = property on="Stop Test Button" class="Bool"("DisabledEnum"=T11."Enabled" ("Disabled")) -> ()  [unwired: 2 in, 2 out]
                n169 = Enqueue Element(queue=w238, element=Control_3."start test" ("Enum")) -> ()  [unwired: 2 in, 3 out]
              }
            }
          }
        }
      }
      event "Log Test Button": Value Change {
        n170 = event-data() -> ()  [unwired: 1 in, 6 out]
        n171 = property on="File Name" class="Str (strict)"() -> ("Value"=w244:T5)  [unwired: 2 in, 2 out]
        n172 = String Length(string=w244) -> (length=w243:i32)
        n173 = Equal To 0?(x=w243) -> (x = 0?=w242:bool)
        n174 = case shown="True" w242 {
          frame False {
          }
          frame True {
            n175 = One Button Dialog(message="A filename has not been entered!") -> ()  [unwired: 1 in, 1 out]
          }
        }
      }
      event "Stop Test Button": Value Change {
        n176 = event-data() -> ()  [unwired: 1 in, 5 out]
        n177 = flat-sequence {
          tunnel: w251 -> [w253]
          tunnel: [w253] -> w250
          tunnel: [w252] -> w248
          tunnel: w250 -> [w257]
          tunnel: [w256] -> w249
          tunnel: w248 -> [w256]
          tunnel: [w255] -> w247
          tunnel: w249 -> [w261]
          tunnel: w247 -> [w260]
          tunnel: [T11."Disabled and Grayed Out" ("Disabled")] -> w246
          frame #0 {
            n178 = local read "Connected?"() -> (w252:bool)
            n179 = local write "Stop Cmd"(T1 1.0 ("Stop Cmd")) -> ()
          }
          frame #1 {
            n180 = Enqueue Element(queue=w257, element=Control_3."main" ("Enum")) -> (queue out=w255:refnum<queue>)  [unwired: 2 in, 2 out]
          }
          frame #2 {
            n181 = case shown="True" w261 {
              tunnel: w260 -> [w262 w265]
              tunnel: [w262 w264] -> _
              frame False {
              }
              frame True {
                n182 = local write "Connected?"(FALSE ("Connected?")) -> ()
                n183 = Enqueue Element(queue=w265, element=Control_3."Multigas disconnect" ("Enum")) -> (queue out=w264:refnum<queue>)  [unwired: 2 in, 2 out]
              }
            }
          }
        }
        n184 = property on="Stop Test Button" class="Bool"("DisabledEnum"=w246) -> ()  [unwired: 2 in, 2 out]
      }
      event "Stopped?": Value Change {
        n185 = event-data() -> ()  [unwired: 1 in, 5 out]
        n186 = flat-sequence {
          tunnel: w269 -> [w273]
          tunnel: [w272] -> w268
          tunnel: [w271] -> w267
          tunnel: w268 -> [w275]
          tunnel: w267 -> [w274]
          frame #0 {
            n187 = local read "Connected?"() -> (w271:bool)
            n188 = Enqueue Element(queue=w273, element=Control_3."main" ("Enum")) -> (queue out=w272:refnum<queue>)  [unwired: 2 in, 2 out]
          }
          frame #1 {
            n189 = case shown="True" w274 {
              tunnel: w275 -> [_ w276]
              frame False {
              }
              frame True {
                n190 = local write "Connected?"(FALSE ("Connected?")) -> ()
                n191 = Enqueue Element(queue=w276, element=Control_3."Multigas disconnect" ("Enum")) -> ()  [unwired: 2 in, 3 out]
              }
            }
          }
        }
      }
      event "Alarm ack": Value Change {
        # "system alarm - set to off"
        n192 = event-data() -> ()  [unwired: 1 in, 5 out]
        n193 = local write "Acknowledge"(TRUE ("Acknowledge")) -> ()
        n194 = property on="Soft Alarm" class="Bool (strict)"("Value"=FALSE ("Acknowledge")) -> ()  [unwired: 2 in, 2 out]
        n195 = property on="Alarm ack" class="Bool"("DisabledEnum"=T11."Disabled and Grayed Out" ("Disabled")) -> ()  [unwired: 2 in, 2 out]
      }
      event "Purge System": Value Change {
        n196 = event-data() -> ()  [unwired: 1 in, 5 out]
        n197 = flat-sequence {
          tunnel: w283 -> [w285]
          tunnel: [w285] -> w282
          tunnel: w282 -> [w286]
          frame #0 {
            n198 = local write "Enum 1"(u16 4 ("Test number")) -> ()
          }
          frame #1 {
            n199 = Enqueue Element(queue=w286, element=Control_3."start test" ("Enum")) -> ()  [unwired: 2 in, 3 out]
          }
        }
      }
      event "Clear log": Value Change {
        n200 = event-data() -> ()  [unwired: 1 in, 5 out]
        n201 = local write "Table"(string[][] [] ("Table")) -> ()
      }
      event "Advanced settings": Value Change {
        # "To be updated"
        # "SO2 conc\nNOx conc\nCO conc\nHC conc\nBleed ratio N2\nBleed ratio CO2"
        n202 = event-data() -> ()  [unwired: 1 in, 5 out]
        n203 = call "Advanced settings MAX.vi"() -> ("output cluster"=→"output cluster":T2)  [unwired: 1 in]
      }
    }
    "stop 2" <- w39
  }
  n204 = node-c288() -> (w2:T12)  [unwired: 4 in]
  n205 = node-c288(nitl_modes."Discard missed periods, maintain original phase" ("Mode")) -> (w9:T12)  [unwired: 4 in]
  n206 = timed-loop {
    timing: w2 -> [_]
    timing-out: [_] -> w1
    stop <- _ stop-if-true
    n207 = node-c288() -> ()  [unwired: 1 in, 1 out]
    n208 = shared-variable "cRIO-9082\\Library 1.lvlib\\DATA_2"() -> (w300:dbl[])  [unwired: 1 in, 1 out]
    n209 = for {
      tunnel: w300 -> [w307] mode=indexing
      tunnel: [w306] -> w292 mode=indexing
      n210 = Number To Fractional String(number=w307, precision (6)=i16 3) -> (F-format string=w306:string)  [unwired: 2 in]
    }
    n211 = Get Date/Time In Seconds() -> (seconds since 1Jan1904=w295:timestamp)
    n212 = local read "File name"() -> (w299:string)
    n213 = Format Date/Time String(time format string (%c)="%d/%m/%y %H:%M:%S", seconds (now)=w295) -> (date/time string=w293:string)  [unwired: 1 in]
    n214 = Concatenate Strings(w299, "_MFC" ("string")) -> (w297:string)
    n215 = Build Array (concatenate)(w293, w292) -> (w291:string[])
    n216 = String To Path(string=w297) -> (path=w294:path)
    n217 = local read "Log?"() -> (w290:bool)
    n218 = case shown="True" w290 {
      tunnel: w294 -> [w301 w304]
      tunnel: [w301 w302] -> _
      tunnel: w291 -> [_ w303]
      frame False {
      }
      frame True {
        n219 = call-poly <vilib>:"Write To Spreadsheet File.vi"("append to file? (new file:F)"=TRUE, "1D data"=w303, "file path (dialog if empty)"=w304) -> ("new file path (Not A Path if cancelled)"=w302:path)  [unwired: 5 in]
      }
    }
    n220 = node-c288() -> ()  [unwired: 1 in, 1 out]
  }
  n221 = timed-loop {
    timing: w9 -> [_]
    timing-out: [_] -> w8
    shift-right: [w313] -> _
    shift-left: path "" -> [w455]
    shift-right: [w413] -> _
    shift-left: w3 -> [w454]
    shift-right: [w314] -> _
    shift-left: _ -> [w424]
    shift-right: [w403] -> _
    shift-left: w3 -> [w406]
    shift-right: [w404] -> _
    shift-left: w3 -> [w405]
    stop <- w453 stop-if-true
    w324 = 54321.0 ("y")
    # "0 Flow Rate 1\n1 Flow Rate 2\n2 CO2 U\n3 CO U\n4 HC U\n5 O2 U\n7 CO2 D\n8 CO D\n9 HC D\n10 O2 D\n12 TC1X\n13 TC2A\n14 TC3Y\n15 TC4B\n16 TC5\n17 TC6\n32 Venturi 1\n33 Venturi 2\n34 Tank\n35 Bearing 1\n36 Bearing 2\n38 Ex A\n39 Ex B\n40 Ex C\n41 Ex D\n42 Furnace 1\n43 Furnace 2\n44 NO 1 ?? \n45 Lambda 1\n46 NO 2 ??\n47 Lambda 2"
    # "ECM AFR"
    n222 = node-c288() -> (→"Finished Late? [i-1]":bool, →"Iteration Duration":i64)  [unwired: 1 in, 1 out]
    n223 = shared-variable "cRIO-9082\\Library 1.lvlib\\DATA"() -> (w452:dbl[])  [unwired: 1 in, 1 out]
    n224 = local read "MKS 1"() -> (w334:i16)
    n225 = local read "MKS 2"() -> (w333:i16)
    n226 = case shown="1" w333 {
      tunnel: [dbl[] [54321.0] w534] -> w330
      frame 0, Default {
      }
      frame 1 {
        # "Connecting to MKS Analyser 2"
        n227 = call "tw_PollRequest simple version.vi"("EVID list"=i32[] [2000, 2001, 2002, 2003, 2004, 2005, 2006, 2007, 2008, 2009, 2010, 2011, 2012, 2013, 2014], "IP_ADD [127.0.0.1]"="192.168.254.2") -> ("values out"=w532:string[])  [unwired: 7 in, 2 out]
        n228 = for {
          tunnel: [w536] -> w530 mode=indexing
          tunnel: w532 -> [w535] mode=indexing
          n229 = Fract/Exp String To Number(string=w535) -> (number=w536:dbl)  [unwired: 3 in, 1 out]
        }
        n230 = Build Array (concatenate)(w530) -> (w534:dbl[])
      }
    }
    n231 = case shown="1" w334 {
      tunnel: [dbl[] [54321.0] w538] -> w332
      frame 0, Default {
      }
      frame 1 {
        # "Connecting to MKS Analyser 1"
        n232 = call "tw_PollRequest simple version.vi"("EVID list"=i32[] [2000, 2001, 2002, 2003, 2004, 2005, 2006, 2007, 2008, 2009, 2010, 2011, 2012, 2013, 2014], "IP_ADD [127.0.0.1]"="192.168.254.1") -> ("values out"=w541:string[])  [unwired: 7 in, 2 out]
        n233 = for {
          tunnel: [w544] -> w539 mode=indexing
          tunnel: w541 -> [w543] mode=indexing
          n234 = Fract/Exp String To Number(string=w543) -> (number=w544:dbl)  [unwired: 3 in, 1 out]
        }
        n235 = Build Array (concatenate)(w539) -> (w538:dbl[])
      }
    }
    n236 = Type Cast(type=w452, x=w452) -> (*(type *) &x=w463:dbl[])
    n237 = local read "Advanced Logging"() -> (w319:bool)
    n238 = Delete From Array(array=w463, length=4, index=0) -> (deleted portion=w460:dbl[], array with subset deleted=w320:dbl[])
    n239 = case shown="True" w319 {
      tunnel: [w484 w505] -> w321
      tunnel: w320 -> [w494 w505]
      tunnel: ["Time\tFlow 1 g/s\tFlow 2 g/s\tECM AFR\tCO2 U %\tCO U %\tHC U ppm\tO2 U %\tNO U ppm\tCO2 D %\tCO D %\tHC D ppm\tO2 D %\tNO D ppm\tTC1X\tTC2A\tTCY\tTC4B\tTC5\tTC6\tTC7\tTC8\tRapidox\tLambda 1\tLambda 2\tNOX 1 ppm\tNOX 2 ppm\tUEGO 1\tUEGO 2" ("Heading string 2") "Time\tFlow 1 g/s\tFlow 2 g/s\tECM AFR\tCO2 U %\tCO U %\tHC U ppm\tO2 U %\tNO U ppm\tCO2 D %\tCO D %\tHC D ppm\tO2 D %\tNO D ppm\tTC1X\tTC2A\tTCY\tTC4B\tTC5\tTC6\tTC7\tTC8\tTC9\tTC10\tTC11\tTC12\tTC13\tTC14\tTC15\tTC16\tTC17\tTC18\tTC19\tTC20\tTC Vent 1\tTC Vent 2\tTC Tank\tTC Fan B1\tTC Fan B2\tTC Cab\tTC Ex A\tTC Ex B\tTC Ex C\tTC Ex D\tTC MFC Box\tTC Furn 1\tTC Furn 2\tTank Pressure\tRapidox\tLambda 1\tLambda 2\tNOX 1 ppm\tNOX 2 ppm\tUEGO 1\tUEGO 2" ("Heading string 2")] -> w318
      frame False {
        n240 = Delete From Array(array=w494, length=21, index=0) -> (deleted portion=w485:dbl[], array with subset deleted=w493:dbl[])
        n241 = Index Array(array=w493, index #1=47 ("index"), index #2=48 ("index"), index #3=49 ("index"), index #4=50 ("index"), index #5=51 ("index"), index #6=52 ("index"), index #7=53 ("index")) -> (element #1=w492:dbl, element #2=w491:dbl, element #3=w490:dbl, element #4=w489:dbl, element #5=w488:dbl, element #6=w487:dbl, element #7=w486:dbl)
        n242 = Build Array (concatenate)(w485, w492, w491, w490, w489, w488, w487, w486) -> (w484:dbl[])
      }
      frame True {
        (unwired) "Time\tFlow 1 g/s\tFlow 2 g/s\tECM AFR\tCO2 U %\tCO U %\tHC U ppm\tO2 U %\tNO U ppm\tCO2 D %\tCO D %\tHC D ppm\tO2 D %\tNO D ppm\tTC1X\tTC2A\tTCY\tTC4B\tTC5\tTC6\tTC7\tTC8\tTC9\tTC10\tTC11\tTC12\tTC13\tTC14\tTC15\tTC16\tTC17\tTC18\tTC19\tTC20\tTC Vent 1\tTC Vent 2\tTC Fan B1\tTC Fan B2\tTC Cab\tTC Ex A\tTC Ex B\tTC Ex C\tTC Ex D\tTC Furn 1\tTC Furn 2\tNOX 1 ppm\tNLambda 1\tNOX 2 ppm\tNLambda 2\tEGO 1\tEGO 2\tEGO 3\tEGO 4\tCO2 U %\tCO U %\tHC U ppm\tO2 U %\tNO U ppm\tCO2 D %\tCO D %\tHC D ppm\tO2 D %\tNO D ppm\r\n" ("Heading string 2")
      }
    }
    n243 = Index Array(array=w460) -> (element #1=w314:dbl, element #2=w430:dbl, element #3=w316:dbl, element #4=w423:dbl)  [unwired: 4 in]
    "Error" <- w316
    n244 = To Unsigned Long Integer(number=w423) -> (unsigned 32bit integer=w422:u32)
    n245 = Number To Boolean Array(number=w422) -> (Boolean array=w442:bool[])
    n246 = Index Array(array=w442) -> (element #2=w440:bool, element #3=w439:bool, element #4=w419:bool)  [unwired: 4 in, 1 out]
    "Extractor Fan On" <- w419
    n247 = case shown="2" w430 {
      tunnel: [w564 TRUE FALSE] -> w429
      tunnel: [w565 FALSE TRUE] -> w428
      frame 0, Default {
        n248 = local read "Pass"() -> (w565:bool)
        n249 = local read "Fail"() -> (w564:bool)
      }
      frame 1 {
      }
      frame 2 {
      }
    }
    "Pass" <- w428
    "Fail" <- w429
    n250 = Or(x=w440, y=w439) -> (x .or. y?=→"Doors Open":bool)
    n251 = Not(x=w419) -> (.not. x?=→"Doors Unlocked":bool)
    n252 = Less?(x=w314, y=w424) -> (x < y?=w421:bool)
    n253 = Path To String(path="File Path") -> (string=w417:string)
    n254 = Index Array(array=w332, index=0) -> (element=w328:dbl)
    n255 = Index Array(array=w330, index=0) -> (element=w326:dbl)
    n256 = local read "Connected"() -> (w420:bool)
    n257 = Concatenate Strings(w417, "\\" ("string"), "File Name") -> (w335:string)
    n258 = Not Equal?(x=w328, y=w324) -> (x != y?=w327:bool)
    n259 = Not Equal?(x=w324, y=w326) -> (x != y?=w325:bool)
    n260 = case shown="True" w327 {
      tunnel: [w511 w522] -> w323
      tunnel: w330 -> [w510 w521]
      tunnel: w332 -> [_ w520]
      tunnel: w325 -> [w509 w519]
      tunnel: [w508 w516] -> w322
      frame False {
        n261 = case shown="False" w509 {
          tunnel: [dbl[] [54321.0] w515] -> w511
          tunnel: w510 -> [_ w515]
          tunnel: ["\r" ("Heading string 2") "\tNO\tNO2 (150)\tNO2 (2000)\tN2O\tNH3 (300)\tNH3 (3000)\tHNCO (400)\tH2O\tCO2\tCO (500)\tCO (1)\tCH4 (250)\tCH4 (3000)\tNOxP\tPropane\r" ("Heading string 2")] -> w506
          frame False {
          }
          frame True {
          }
        }
        n262 = Build Array(" " ("Heading string 2"), w506) -> (w508:string[])
      }
      frame True {
        n263 = case shown="True" w519 {
          tunnel: [w524 w528] -> w522
          tunnel: w521 -> [_ w527]
          tunnel: w520 -> [w524 w526]
          tunnel: ["\rn" ("Heading string 2") "\tNO\tNO2 (150)\tNO2 (2000)\tN2O\tNH3 (300)\tNH3 (3000)\tHNCO (400)\tH2O\tCO2\tCO (500)\tCO (1)\tCH4 (250)\tCH4 (3000)\tNOxP\tPropane\r" ("Heading string 2")] -> w517
          frame False {
          }
          frame True {
            n264 = Build Array (concatenate)(w526, w527) -> (w528:dbl[])
          }
        }
        n265 = Build Array("\tNO\tNO2 (150)\tNO2 (2000)\tN2O\tNH3 (300)\tNH3 (3000)\tHNCO (400)\tH2O\tCO2\tCO (500)\tCO (1)\tCH4 (250)\tCH4 (3000)\tNOxP\tPropane" ("Heading string 2"), w517) -> (w516:string[])
      }
    }
    n266 = And(x=w420, y=w421) -> (x .and. y?=w412:bool)
    n267 = local write "Stopped?"(w412) -> ()
    n268 = Equal To 0?(x=w316) -> (x = 0?=w317:bool)
    n269 = Equal To 0?(x=w314) -> (x = 0?=w315:bool)
    n270 = Build Array (concatenate)(w321, w323) -> (w456:dbl[])
    n271 = Equal?(x=w314, y=2.0) -> (x = y?=w348:bool)
    n272 = String To Path(string=w335) -> (path=w414:path)
    n273 = Build Array(w317, w315) -> (w436:bool[])
    n274 = Equal?(x=w314, y=3.0) -> (x = y?=w340:bool)
    n275 = Equal?(x=w314, y=4.0) -> (x = y?=w338:bool)
    n276 = Boolean Array To Number(Boolean array=w436) -> (number=w435:u32)
    n277 = Not Equal?(x=w414, y=w455) -> (x != y?=w465:bool)
    n278 = Compound Arithmetic op=OR(w348, w340, w338) -> (w347:bool)
    n279 = local read "Log Test Button"() -> (w336:bool)
    n280 = case shown="1" w435 {
      tunnel: [w589 w590 w595 w597] -> w437
      tunnel: [w589 w590 w595 w597] -> w434
      tunnel: [w589 w590 w595 w597] -> w433
      tunnel: [w589 w590 w593 w597] -> w432
      tunnel: [T11."Enabled" ("Disabled") T11."Enabled" ("Disabled") w593 w597] -> w431
      tunnel: [FALSE FALSE FALSE TRUE] -> w411
      frame 0, Default {
        w589 = T11."Disabled and Grayed Out" ("Disabled")
      }
      frame 1 {
        w590 = T11."Disabled and Grayed Out" ("Disabled")
      }
      frame 2 {
        w593 = T11."Enabled" ("Disabled")
        w595 = T11."Disabled and Grayed Out" ("Disabled")
      }
      frame 3 {
        w597 = T11."Enabled" ("Disabled")
        (unwired) T11."Disabled and Grayed Out" ("Disabled")
      }
    }
    n281 = for {
      tunnel: w456 -> [w605] mode=indexing
      tunnel: [w604] -> w467 mode=indexing
      n282 = Number To Fractional String(number=w605, precision (6)=i16 3) -> (F-format string=w604:string)  [unwired: 2 in]
    }
    n283 = Select(t=w414, s=w465, f=w455) -> (s? t:f=w466:path)
    n284 = case shown="True" w465 {
      tunnel: w466 -> [w598 w603]
      tunnel: [w598 w602] -> w464
      tunnel: w322 -> [_ w600]
      tunnel: w318 -> [_ w599]
      frame False {
      }
      frame True {
        # "setting up the header"
        n285 = Build Array (concatenate)(w599, w600) -> (w601:string[])
        n286 = call-poly <vilib>:"Write To Spreadsheet File.vi"("1D data"=w601, "file path (dialog if empty)"=w603) -> ("new file path (Not A Path if cancelled)"=w602:path)  [unwired: 6 in]
      }
    }
    n287 = And(x=w336, y=w347) -> (x .and. y?=w482:bool)
    "Log?" <- w482
    n288 = Equal?(x=w314, y=0.0) -> (x = y?=w400:bool)
    n289 = case shown="5" w314 {
      tunnel: [w551 w554 w556 w558 TRUE FALSE] -> w427
      tunnel: [w551 TRUE TRUE TRUE w560 w562] -> w426
      tunnel: [TRUE w554 w556 w558 w560 w562] -> w425
      frame 0, Default {
        w551 = FALSE
      }
      frame 1 {
        w554 = FALSE
      }
      frame 2 {
        w556 = FALSE
      }
      frame 3 {
        w558 = FALSE
      }
      frame 4 {
        w560 = FALSE
        n290 = local write "Stop Cmd"(T1 0.0 ("Stop Cmd")) -> ()
      }
      frame 5 {
        w562 = FALSE
      }
    }
    "Cool Down" <- w427
    "Test In Progress" <- w426
    "Standby" <- w425
    n291 = property on="Start Test Button" class="Bool"("DisabledEnum"=w437) -> ()  [unwired: 2 in, 2 out]
    n292 = property on="Execute Leak Test Button" class="Bool"("DisabledEnum"=w434) -> ()  [unwired: 2 in, 2 out]
    n293 = property on="Compile Test Button" class="Bool"("DisabledEnum"=w433) -> ()  [unwired: 2 in, 2 out]
    n294 = property on="Purge System" class="Bool"("DisabledEnum"=w432) -> ()  [unwired: 2 in, 2 out]
    n295 = property on="Advanced settings" class="Bool"("DisabledEnum"=w431) -> ()  [unwired: 2 in, 2 out]
    n296 = property class="VI"("Front Panel.Closeable"=w411) -> ()  [unwired: 2 in, 2 out]
    n297 = Delete From Array(array=w320, length=1, index=2) -> (deleted portion=w344:dbl[], array with subset deleted=w342:dbl[])
    n298 = Index Array(array=w323, index #1=0 ("index"), index #2=1 ("index"), index #3=2 ("index"), index #4=3 ("index")) -> ()  [unwired: 4 out]
    n299 = Index Array(array=w344) -> (element=w343:dbl)  [unwired: 1 in]
    n300 = local read "Full system?"() -> (w401:bool)
    n301 = Not Equal To 0?(x=w316) -> (x != 0?=w458:bool)
    n302 = Not Equal?(x=w316, y=w454) -> (x != y?=w457:bool)
    n303 = case shown="True" w482 {
      tunnel: w464 -> [w609 w617]
      tunnel: [w609 w629] -> w313
      tunnel: w467 -> [_ w625]
      tunnel: w406 -> [_ w618]
      tunnel: w405 -> [w608 w613]
      tunnel: [w608 w615] -> w404
      tunnel: [w607 w614] -> w403
      frame False {
        n304 = local read "Log interval (seconds)"() -> (w607:T1)
      }
      frame True {
        n305 = Get Date/Time In Seconds() -> (seconds since 1Jan1904=w626:timestamp)
        n306 = Decrement(x=w618) -> (x-1=w619:T1)
        n307 = Less Than 0?(x=w619) -> (x < 0?=w620:bool)
        n308 = Equal To 0?(x=w619) -> (x = 0?=w621:bool)
        n309 = Build Array(w620, w621) -> (w622:bool[])
        n310 = Path To String(path=w617) -> (string=w612:string)
        "File name" <- w612
        n311 = Format Date/Time String(time format string (%c)="%d/%m/%y %H:%M:%S", seconds (now)=w626) -> (date/time string=w627:string)  [unwired: 1 in]
        n312 = Boolean Array To Number(Boolean array=w622) -> (number=w623:u32)
        n313 = case shown="2" w623 {
          tunnel: w618 -> [w636 w637 _]
          tunnel: [w635 w637 w640] -> w614
          tunnel: w612 -> [w634 w639 w643]
          tunnel: [w631 w639 w641] -> w616
          tunnel: [w630 w638 w642] -> w615
          tunnel: w613 -> [w630 w638 w646]
          frame 0, Default {
            n314 = Number To Decimal String(number=w630) -> (decimal integer string=w632:string)  [unwired: 1 in]
            n315 = call <vilib>:"Space Constant.vi"() -> ("String"=w633:string)
            n316 = Decrement(x=w636) -> (x-1=w635:T1)
            n317 = Concatenate Strings(w634, w633, w632) -> (w631:string)
          }
          frame 1 {
          }
          frame 2 {
            n318 = local read "Log interval (seconds)"() -> (w640:T1)
            n319 = Increment(x=w646) -> (x+1=w642:dbl)
            n320 = Number To Decimal String(number=w642) -> (decimal integer string=w644:string)  [unwired: 1 in]
            n321 = call <vilib>:"Space Constant.vi"() -> ("String"=w645:string)
            n322 = Concatenate Strings(w643, w645, w644) -> (w641:string)
          }
        }
        n323 = Build Array (concatenate)(w627, w625) -> (w611:string[])
        n324 = String To Path(string=w616) -> (path=w610:path)
        n325 = call-poly <vilib>:"Write To Spreadsheet File.vi"("append to file? (new file:F)"=TRUE, "1D data"=w611, "file path (dialog if empty)"=w610) -> ("new file path (Not A Path if cancelled)"=w629:path)  [unwired: 5 in]
      }
    }
    n326 = And(x=w458, y=w457) -> (x .and. y?=w459:bool)
    n327 = Index Array(array=w342, index #1=0 ("index"), index #2=1 ("index"), index #3=2 ("index"), index #4=3 ("index"), index #5=4 ("index"), index #6=5 ("index"), index #7=7 ("index"), index #8=8 ("index"), index #9=9 ("index"), index #10=10 ("index"), index #11=12 ("index"), index #12=13 ("index"), index #13=14 ("index"), index #14=15 ("index"), index #15=16 ("index"), index #16=17 ("index"), index #17=32 ("index"), index #18=33 ("index"), index #19=34 ("index"), index #20=35 ("index"), index #21=36 ("index"), index #22=38 ("index"), index #23=39 ("index"), index #24=40 ("index"), index #25=41 ("index"), index #26=43 ("index"), index #27=44 ("index"), index #28=49 ("index"), index #29=50 ("index"), index #30=47 ("index"), index #31=48 ("index")) -> (element #1=w398:dbl, element #2=w397:dbl, element #3=w394:dbl, element #4=w392:dbl, element #5=w393:dbl, element #6=w391:dbl, element #7=w390:dbl, element #8=w389:dbl, element #9=w388:dbl, element #10=w387:dbl, element #11=w382:dbl, element #12=w381:dbl, element #13=w380:dbl, element #14=w379:dbl, element #15=w378:dbl, element #16=w377:dbl, element #17=w371:dbl, element #18=w370:dbl, element #19=w369:dbl, element #20=w368:dbl, element #21=w367:dbl, element #22=w362:dbl, element #23=w361:dbl, element #24=w360:dbl, element #25=w359:dbl, element #26=→"Furnace temp 1":dbl, element #27=→"Furnace temp 2":dbl, element #28=w352:dbl, element #29=w312:dbl, element #30=w311:dbl, element #31=w349:dbl)
    n328 = Build Array(w401, w400) -> (w402:bool[])
    n329 = case shown="True" w459 {
      tunnel: w316 -> [w571 w582]
      tunnel: w457 -> [w574 _]
      tunnel: [w570 w582] -> w413
      frame False {
        n330 = Equal To 0?(x=w571) -> (x = 0?=w575:bool)
        n331 = And(x=w575, y=w574) -> (x .and. y?=w573:bool)
        n332 = case shown="True" w573 {
          frame False {
          }
          frame True {
            w578 = FALSE ("Ack hard alarm!")
            n333 = property on="Hard Alarm" class="Bool (strict)"("Value"=w578) -> ()  [unwired: 2 in, 2 out]
            n334 = property on="System Alarm" class="Bool (strict)"("Value"=w578) -> ()  [unwired: 2 in, 2 out]
          }
        }
        n335 = case shown="False" "Acknowledge" {
          tunnel: [w576 0.0 ("Numeric")] -> w570
          tunnel: w571 -> [w576 _]
          frame False {
          }
          frame True {
          }
        }
      }
      frame True {
        n336 = local read "Table"() -> (w585:string[][])
        n337 = call "Error list.vi"("Error code"=w582, "Error array in"=w585) -> ("Hard alarm?"=w579:bool, "Error array out"=w584:string[][])  [unwired: 8 in]
        "Hard Alarm" <- w579
        "System Alarm" <- w579
        n338 = Not(x=w579) -> (.not. x?=w580:bool)
        "Soft Alarm" <- w580
        n339 = case shown="True" w580 {
          frame False {
          }
          frame True {
            n340 = property on="Alarm ack" class="Bool"("DisabledEnum"=T11."Enabled" ("Disabled")) -> ()  [unwired: 2 in, 2 out]
          }
        }
        n341 = local write "Table"(w584) -> ()
        n342 = local write "Acknowledge"(FALSE ("Acknowledge")) -> ()
        n343 = property on="Tab Control" class="TabCtl (strict)"("Value"=6) -> ()  [unwired: 2 in, 2 out]
      }
    }
    n344 = Boolean Array To Number(Boolean array=w402) -> (number=w399:u32)
    n345 = case shown="1" w399 {
      tunnel: w398 -> [w546 w548 _ _]
      tunnel: w397 -> [_ w547 _ _]
      tunnel: [w546 w548 w549 w550] -> w396
      tunnel: [0.0 ("y") w547 w549 w550] -> w395
      frame 0, Default {
      }
      frame 1 {
      }
      frame 2 {
        w549 = 0.0 ("y")
      }
      frame 3 {
        w550 = 0.0 ("y")
      }
    }
    n346 = Merge Signals(w396, w395) -> (→"Flow Rate (g/s)":dynamicdata)
    n347 = Merge Signals(w394, w392, w391, w390, w389, w387) -> (→"M584L Upstream & Downstream":dynamicdata)
    n348 = Merge Signals(w393, w388) -> (→"HC Concentration (ppm)":dynamicdata)
    n349 = Merge Signals(w382, w381, w380, w379, w378, w377) -> (→"Sample Temperatures (°C)":dynamicdata)
    n350 = Merge Signals(w371, w370, w369, w368, w367) -> (→"System Temperatures (°C)":dynamicdata)
    n351 = Merge Signals(w362, w361, w360, w359) -> (→"Heat Exchanger Temperatures (°C)":dynamicdata)
    n352 = Merge Signals(w352, w312) -> (→"NO Concentration (ppm)":dynamicdata)
    n353 = Merge Signals(w311, w349, w343) -> (→"Lambda":dynamicdata)
    n354 = local read "stop 2"() -> (w453:bool)
    n355 = node-c288() -> ()  [unwired: 1 in, 1 out]
  }
  n356 = while {
    tunnel: w37 -> [w655]
    tunnel: w21 -> [w653]
    tunnel: w23 -> [w652]
    tunnel: [FALSE ("stop 2")] -> w11
    stop <- w656 stop-if-true
    n357 = Dequeue Element(queue=w655) -> (element=w654:T10)  [unwired: 2 in, 3 out]
    n358 = case shown="\"main\", Default" w654 {
      tunnel: w653 -> [_ _ _ w707 w718 w754 w788 _ _ _ _ _ _ _ w1151 _ _ _ _ _ _ _]
      tunnel: w652 -> [_ _ _ _ _ _ _ _ w801 w816 w871 w916 _ _ _ _ _ _ _ _ _ _]
      frame "main", Default {
        # "20"
        # "25"
        # "30"
        # "15"
        # "10"
        # "5"
        # "0"
        # "30"
        # "25"
        # "20"
        # "15"
        # "10"
        # "5"
        # "0"
        # "Output Cluster\n\n0 NOx Conc\n1 CO conc %\n2 HC conc %\n3 Bleed H2O \n4 Bleed CO2\n5 Bleed N2 \n6 lambda P\n7 lambda I\n8 lambda D\n9 purge duration\n10 Target furnace lambda\n11 HC reaction ct\n12 Full system\n13 Log interval\n14 MKS 1\n15 MKS 2"
        n359 = local read "output cluster"() -> (w681:T2)
        n360 = Unbundle(w681) -> ("NOx Concentration (ppm)"=w667:T1, "CO concentration %"=w666:T1, "HC concentration %"=w665:T1, "Bleed H2O %"=w664:T1, "Bleed CO2 %"=w663:T1, "Bleed N2 %"=w678:T1, "lambda P"=w677:T1, "lambda I"=w676:T1, "lambda D"=w679:T1, "Purge duration (seconds)"=w680:T1, "Target furnace lambda"=w672:T1, "HC reaction constant"=w671:T1, w673:i16, "Log interval (HRS)"=→"Log interval (seconds)":T1, w660:i16, w658:i16, "Advanced Logging"=→"Advanced Logging":bool)
        "MKS 1" <- w660
        "MKS 2" <- w658
        n361 = local read "Test Flow Rate(g/s)"() -> (w693:T1)
        n362 = local read "Test number"() -> (w698:u16)
        n363 = local read "Inlet LAMBDA"() -> (w685:T1)
        n364 = local read "NO ppm Loff"() -> (w683:T1)
        n365 = local read "NO:CO Ratio"() -> (w682:T1)
        n366 = local read "Inlet O2 (%)"() -> (w684:T1)
        n367 = local read "Connected"() -> (w687:bool)
        n368 = Boolean To (0,1)(Boolean=w687) -> (0, 1=w670:i16)
        n369 = Not Equal To 0?(x=w660) -> (x != 0?=w661:bool)
        n370 = Not Equal To 0?(x=w658) -> (x != 0?=w659:bool)
        n371 = Or(x=w661, y=w659) -> (x .or. y?=→"Connected":bool)
        n372 = Not Equal To 0?(x=w673) -> (x != 0?=→"Full system?":bool)
        n373 = Build Array("Stop Cmd", w698, w693, "Test Start Temperature (°C)", "Test Stop temperature (°C)", "Furnace Ramp Rate (°C/min)", w685, w684, "Inlet LAMBDA Rich", "Inlet LAMBDA Lean", "Inlet Temperature (°C)", "NO ppm SW", w683, w682, "Temperature Limit (°C)", w670, "Inlet temp Age", "Flow rate Age", w667, w666, w665, w664, w663, w678, w677, w676, w679, w680, w672, w671, w673) -> (w689:T1[])
        n374 = shared-variable "cRIO-9082\\Library 1.lvlib\\Control Variables"(w689) -> ()  [unwired: 1 in, 1 out]
      }
      frame "start test" {
        w699 = FALSE
        n375 = property on="Pass" class="Bool (strict)"("Value"=w699) -> ()  [unwired: 2 in, 2 out]
        n376 = property on="Fail" class="Bool (strict)"("Value"=w699) -> ()  [unwired: 2 in, 2 out]
        n377 = local write "Pass"(w699) -> ()
        n378 = local write "Fail"(w699) -> ()
        n379 = shared-variable "cRIO-9082\\Library 1.lvlib\\Enum 1"("Enum 1") -> ()  [unwired: 1 in, 1 out]
      }
      frame "clear table 1" {
        n380 = property on="Sub-Cycle Name" class="Str (strict)"("Value"="" ("Subcycle name")) -> ()  [unwired: 2 in, 2 out]
        n381 = local write "Flag1"(FALSE) -> ()
        n382 = local write "Sub-Cycle Pattern"(string[][] [["", "0", "", "", "", "", "", "", "", "", "", "", ""], ["", "", "", "", "", "", "", "", "", "", "", "", ""], ["", "", "", "", "", "", "", "", "", "", "", "", ""], ["", "", "", "", "", "", "", "", "", "", "", "", ""], ["", "", "", "", "", "", "", "", "", "", "", "", ""], ["", "", "", "", "", "", "", "", "", "", "", "", ""], ["", "", "", "", "", "", "", "", "", "", "", "", ""], ["", "", "", "", "", "", "", "", "", "", "", "", ""], ["", "", "", "", "", "", "", "", "", "", "", "", ""], ["", "", "", "", "", "", "", "", "", "", "", "", ""], ["", "", "", "", "", "", "", "", "", "", "", "", ""], ["", "", "", "", "", "", "", "", "", "", "", "", ""], ["", "", "", "", "", "", "", "", "", "", "", "", ""], ["", "", "", "", "", "", "", "", "", "", "", "", ""], ["", "", "", "", "", "", "", "", "", "", "", "", ""], ["", "", "", "", "", "", "", "", "", "", "", "", ""], ["", "", "", "", "", "", "", "", "", "", "", "", ""], ["", "", "", "", "", "", "", "", "", "", "", "", ""], ["", "", "", "", "", "", "", "", "", "", "", "", ""], ["", "", "", "", "", "", "", "", "", "", "", "", ""], ["", "", "", "", "", "", "", "", "", "", "", "", ""], ["", "", "", "", "", "", "", "", "", "", "", "", ""], ["", "", "", "", "", "", "", "", "", "", "", "", ""], ["", "", "", "", "", "", "", "", "", "", "", "", ""], ["", "", "", "", "", "", "", "", "", "", "", "", ""], ["", "", "", "", "", "", "", "", "", "", "", "", ""], ["", "", "", "", "", "", "", "", "", "", "", "", ""], ["", "", "", "", "", "", "", "", "", "", "", "", ""], ["", "", "", "", "", "", "", "", "", "", "", "", ""], ["", "", "", "", "", "", "", "", "", "", "", "", ""], ["", "", "", "", "", "", "", "", "", "", "", "", ""]]) -> ()
      }
      frame "update list 1" {
        n383 = String To Path(string=w707) -> (path=w706:path)
        n384 = List Folder(path=w706, pattern="*.eyes") -> (filenames=w705:string[])  [unwired: 2 in, 3 out]
        n385 = property on="Sub-Cycle List" class="LstBox (strict)"("Item Names"=w705) -> ()  [unwired: 2 in, 2 out]
      }
      frame "save subc" {
        w711 = ".eyes" ("string")
        n386 = local read "Sub-Cycle Name"() -> (w710:T5)
        n387 = String To Path(string=w718) -> (path=w723:path)
        n388 = Equal?(x=w710, y="") -> (x = y?=w715:bool)
        n389 = List Folder(path=w723, pattern="*.eyes" ("string")) -> (filenames=w722:string[])  [unwired: 2 in, 3 out]
        n390 = Concatenate Strings(w710, w711) -> (w709:string)
        n391 = Concatenate Strings(w718, w710, w711) -> (w724:string)
        n392 = Search 1D Array(1D array=w722, element=w709) -> (index of element=w721:i32)  [unwired: 1 in]
        n393 = case shown="True" w715 {
          tunnel: [TRUE FALSE] -> w714
          frame False {
          }
          frame True {
            n394 = One Button Dialog(message="Insert file name!") -> ()  [unwired: 1 in, 1 out]
          }
        }
        n395 = String To Path(string=w724) -> (path=w717:path)
        n396 = Equal?(x=w721, y=-1) -> (x = y?=w719:bool)
        n397 = case shown="False" w719 {
          selector: w719 -> [_ w730]
          tunnel: [w728 w730] -> w713
          frame False {
            n398 = Two Button Dialog(message="A file with this name already exists!\nDo you want to overwrite?") -> (T button?=w728:bool)  [unwired: 2 in]
          }
          frame True {
          }
        }
        n399 = And(x=w713, y=w714) -> (x .and. y?=w712:bool)
        n400 = case shown="True" w712 {
          tunnel: w717 -> [_ w735]
          frame False {
          }
          frame True {
            n401 = local read "Sub-Cycle Pattern"() -> (w734:string[][])
            n402 = call "Table check.vi"("Input table"=w734) -> ("Incomplete?"=w732:bool, "Length"=w733:i32)  [unwired: 9 in]
            n403 = case shown="False" w732 {
              tunnel: w734 -> [w743 _]
              tunnel: w735 -> [w742 _]
              tunnel: w733 -> [w741 _]
              tunnel: string[] [] -> [w740 _]
              frame False {
                n404 = for {
                  N: w741 -> [_]
                  tunnel: w743 -> [w750]
                  shift-right: [w747] -> w739
                  shift-left: w740 -> [w748]
                  i -> [w749]
                  n405 = Index Array(array=w750, index (row)=w749) -> (element=w746:string[])  [unwired: 1 in]
                  n406 = Delete From Array(array=w746, index=0) -> (array with subset deleted=w745:string[])  [unwired: 1 in, 1 out]
                  n407 = Build Array (concatenate)(w748, w745) -> (w747:string[])
                }
                n408 = Build Array (concatenate)("SubCycle Data File for EYECAT - do not modify", w739) -> (w737:string[])
                n409 = call-poly <vilib>:"Write To Spreadsheet File.vi"("1D data"=w737, "file path (dialog if empty)"=w742) -> ()  [unwired: 6 in, 1 out]
              }
              frame True {
                n410 = One Button Dialog(message="The table is incomplete!\nplease review and save again!") -> ()  [unwired: 1 in, 1 out]
              }
            }
            n411 = local write "Flag1"(FALSE) -> ()
          }
        }
      }
      frame "load subc" {
        n412 = local read "Flag1"() -> (w755:bool)
        n413 = case shown="True" w755 {
          tunnel: [w782 w784] -> w753
          tunnel: w754 -> [w782 w784]
          tunnel: [TRUE w783] -> w752
          frame False {
          }
          frame True {
            n414 = Two Button Dialog(message="The table has been modified.\nDo you want to continue?") -> (T button?=w783:bool)  [unwired: 2 in]
          }
        }
        n415 = case shown="True" w752 {
          tunnel: w753 -> [_ w759]
          frame False {
          }
          frame True {
            n416 = property on="Sub-Cycle List" class="LstBox (strict)"() -> ("Item Names"=w771:string[])  [unwired: 2 in, 2 out]
            n417 = Index Array(array=w771, index="Sub-Cycle List") -> (element=w758:string)
            n418 = Concatenate Strings(w759, w758) -> (w769:string)
            n419 = Search/Split String(string=w758, search string/char (-)=".") -> (substring before match=w756:string)  [unwired: 1 in, 2 out]
            n420 = local write "Sub-Cycle Name"(w756) -> ()
            n421 = String To Path(string=w769) -> (path=w768:path)
            n422 = call-poly <vilib>:"Read From Spreadsheet File.vi"("file path (dialog if empty)"=w768) -> ("first row"=w764:string[])  [unwired: 6 in, 4 out]
            n423 = Delete From Array(array=w764, length=1, index=0) -> (array with subset deleted=w761:string[])  [unwired: 1 out]
            n424 = Array Size(array=w761) -> (size(s)=w767:i32)
            n425 = Divide(x=w767, y=12) -> (x/y=w760:dbl)
            n426 = for {
              N: w760 -> [_]
              shift-right: [w777] -> _
              shift-left: w761 -> [w780]
              tunnel: [w776] -> w765 mode=indexing
              i -> [w775]
              n427 = Increment(x=w775) -> (x+1=w774:i32)
              n428 = Delete From Array(array=w780, length=12, index=0) -> (deleted portion=w772:string[], array with subset deleted=w777:string[])
              n429 = Number To Decimal String(number=w774) -> (decimal integer string=w773:string)  [unwired: 1 in]
              n430 = Build Array (concatenate)(w773, w772) -> (w776:string[])
            }
            n431 = local write "Sub-Cycle Pattern"(w765) -> ()
          }
        }
      }
      frame "delete subc" {
        n432 = Two Button Dialog(message="This operation will permanently delete this file!\nDo you want to continue?") -> (T button?=w787:bool)  [unwired: 2 in]
        n433 = case shown="True" w787 {
          tunnel: w788 -> [_ w793]
          frame False {
          }
          frame True {
            n434 = local read "Sub-Cycle List"() -> (w790:i32)
            n435 = property on="Sub-Cycle List" class="LstBox (strict)"() -> ("Item Names"=w791:string[])  [unwired: 2 in, 2 out]
            n436 = Index Array(array=w791, index=w790) -> (element=w795:string)
            n437 = Concatenate Strings(w793, w795) -> (w794:string)
            n438 = local write "Flag1"(FALSE) -> ()
            n439 = String To Path(string=w794) -> (path=w792:path)
            n440 = Delete(path (use dialog)=w792) -> ()  [unwired: 4 in, 3 out]
          }
        }
      }
      frame "clear table 2" {
        n441 = property on="Cycle Name" class="Str (strict)"("Value"="" ("Subcycle name")) -> ()  [unwired: 2 in, 2 out]
        n442 = local write "Flag 2"(FALSE) -> ()
        n443 = local write "Cycle Pattern"(string[][] [["", "", "", "", ""], ["", "", "", "", ""], ["", "", "", "", ""], ["", "", "", "", ""], ["", "", "", "", ""], ["", "", "", "", ""], ["", "", "", "", ""], ["", "", "", "", ""], ["", "", "", "", ""], ["", "", "", "", ""], ["", "", "", "", ""], ["", "", "", "", ""], ["", "", "", "", ""], ["", "", "", "", ""], ["", "", "", "", ""], ["", "", "", "", ""], ["", "", "", "", ""], ["", "", "", "", ""], ["", "", "", "", ""], ["", "", "", "", ""], ["", "", "", "", ""], ["", "", "", "", ""], ["", "", "", "", ""], ["", "", "", "", ""], ["", "", "", "", ""], ["", "", "", "", ""], ["", "", "", "", ""], ["", "", "", "", ""], ["", "", "", "", ""], ["", "", "", "", ""], ["", "", "", "", ""]]) -> ()
      }
      frame "update list 2" {
        n444 = String To Path(string=w801) -> (path=w802:path)
        n445 = List Folder(path=w802, pattern="*.eyec") -> (filenames=w800:string[])  [unwired: 2 in, 3 out]
        n446 = property on="Cycle List" class="LstBox (strict)"("Item Names"=w800) -> ()  [unwired: 2 in, 2 out]
      }
      frame "save cycle" {
        w803 = ".eyec" ("string")
        n447 = local read "Cycle Name"() -> (w804:T5)
        n448 = String To Path(string=w816) -> (path=w817:path)
        n449 = List Folder(path=w817, pattern="*.eyec" ("string")) -> (filenames=w815:string[])  [unwired: 2 in, 3 out]
        n450 = Equal?(x=w804, y="") -> (x = y?=w810:bool)
        n451 = Concatenate Strings(w804, w803) -> (w806:string)
        n452 = Search 1D Array(1D array=w815, element=w806) -> (index of element=w814:i32)  [unwired: 1 in]
        n453 = Concatenate Strings(w816, w804, w803) -> (w819:string)
        n454 = case shown="True" w810 {
          tunnel: [TRUE FALSE] -> w808
          frame False {
          }
          frame True {
            n455 = One Button Dialog(message="Insert file name!") -> ()  [unwired: 1 in, 1 out]
          }
        }
        n456 = String To Path(string=w819) -> (path=w818:path)
        n457 = Equal?(x=w814, y=-1) -> (x = y?=w812:bool)
        n458 = case shown="False" w812 {
          selector: w812 -> [_ w868]
          tunnel: [w866 w868] -> w809
          frame False {
            n459 = Two Button Dialog(message="A file with this name already exists!\nDo you want to overwrite?") -> (T button?=w866:bool)  [unwired: 2 in]
          }
          frame True {
          }
        }
        n460 = And(x=w809, y=w808) -> (x .and. y?=w807:bool)
        n461 = case shown="True" w807 {
          tunnel: w818 -> [_ w826]
          frame False {
          }
          frame True {
            n462 = local read "Cycle Pattern"() -> (w825:string[][])
            n463 = call "Table check.vi"("Input table"=w825) -> ("Incomplete?"=w823:bool, "Length"=w824:i32)  [unwired: 9 in]
            n464 = case shown="False" w823 {
              tunnel: w826 -> [w835 _]
              tunnel: w825 -> [w834 _]
              tunnel: w824 -> [w827 _]
              frame False {
                n465 = Number To Decimal String(number=w827) -> (decimal integer string=w830:string)  [unwired: 1 in]
                n466 = for {
                  N: w827 -> [_]
                  tunnel: w834 -> [w864]
                  shift-right: [w852] -> w831
                  shift-left: string[] [] -> [w862]
                  i -> [w863]
                  w843 = 12 ("length")
                  n467 = Index Array(array=w864, index (row)=w863) -> (element=w858:string[])  [unwired: 1 in]
                  n468 = Index Array(array=w858, index=3) -> (element=w848:string)
                  n469 = Index Array(array=w858, index=1) -> (element=w847:string)
                  n470 = Concatenate Strings("C:\\Setup Files\\Subcycles Folder\\", w847) -> (w859:string)
                  n471 = String To Path(string=w859) -> (path=w860:path)
                  n472 = call-poly <vilib>:"Read From Spreadsheet File.vi"("file path (dialog if empty)"=w860) -> ("first row"=w851:string[])  [unwired: 6 in, 4 out]
                  n473 = Delete From Array(array=w851, length=1, index=0) -> (array with subset deleted=w845:string[])  [unwired: 1 out]
                  n474 = String Length(string=w845) -> (length=w854:i32[])
                  n475 = Array Size(array=w854) -> (size(s)=w846:i32)
                  n476 = Divide(x=w846, y=w843) -> (x/y=w844:dbl)
                  n477 = Decrement(x=w844) -> (x-1=w836:dbl)
                  n478 = Multiply(x=w843, y=w836) -> (x*y=w842:dbl)
                  n479 = Number To Decimal String(number=w836) -> (decimal integer string=w853:string)  [unwired: 1 in]
                  n480 = Delete From Array(array=w845, length=12, index=w842) -> (deleted portion=w839:string[], array with subset deleted=w840:string[])
                  n481 = Index Array(array=w839, index=0) -> (element=w837:string)
                  n482 = Build Array (concatenate)(w847, w848, w853, w837, w840) -> (w857:string[])
                  n483 = Build Array (concatenate)(w862, w857) -> (w852:string[])
                }
                n484 = local write "Flag 2"(FALSE) -> ()
                n485 = Build Array (concatenate)("Cycle Data File for EYECAT - do not modify", w830, w831) -> (w832:string[])
                n486 = call-poly <vilib>:"Write To Spreadsheet File.vi"("1D data"=w832, "file path (dialog if empty)"=w835) -> ()  [unwired: 6 in, 1 out]
              }
              frame True {
                n487 = One Button Dialog(message="The table is incomplete!\nplease review and save again!") -> ()  [unwired: 1 in, 1 out]
              }
            }
          }
        }
      }
      frame "load cycle" {
        n488 = local read "Flag 2"() -> (w872:bool)
        n489 = case shown="True" w872 {
          tunnel: [w911 w913] -> w869
          tunnel: w871 -> [w911 w913]
          tunnel: [TRUE ("T button?") w912] -> w870
          frame False {
          }
          frame True {
            n490 = Two Button Dialog(message="The table has been modified.\nDo you want to continue?") -> (T button?=w912:bool)  [unwired: 2 in]
          }
        }
        n491 = case shown="True" w870 {
          tunnel: w869 -> [_ w875]
          frame False {
          }
          frame True {
            n492 = property on="Cycle List" class="LstBox (strict)"() -> ("Item Names"=w891:string[])  [unwired: 2 in, 2 out]
            n493 = Index Array(array=w891, index="Cycle List") -> (element=w877:string)
            n494 = Concatenate Strings(w875, w877) -> (w890:string)
            n495 = Search/Split String(string=w877, search string/char (-)=".") -> (substring before match=w876:string)  [unwired: 1 in, 2 out]
            n496 = String To Path(string=w890) -> (path=w889:path)
            n497 = local write "Cycle Name"(w876) -> ()
            n498 = call-poly <vilib>:"Read From Spreadsheet File.vi"("file path (dialog if empty)"=w889) -> ("first row"=w873:string[])  [unwired: 6 in, 4 out]
            n499 = Delete From Array(array=w873, length=2, index=0) -> (array with subset deleted=w874:string[])  [unwired: 1 out]
            n500 = Index Array(array=w873, index=1) -> (element=w888:string)
            n501 = Decimal String To Number(string=w888) -> (number=w887:i32)  [unwired: 2 in, 1 out]
            n502 = for {
              N: w887 -> [_]
              tunnel: w874 -> [w909]
              tunnel: [w904] -> w882 mode=indexing
              shift-right: [w894] -> _
              shift-left: 0 ("x") -> [w895]
              i -> [w908]
              w905 = ""
              n503 = Increment(x=w895) -> (x+1=w893:i32)
              n504 = Increment(x=w893) -> (x+1=w901:i32)
              n505 = Increment(x=w908) -> (x+1=w903:i32)
              n506 = Number To Decimal String(number=w903) -> (decimal integer string=w902:string)  [unwired: 1 in]
              n507 = Index Array(array=w909, index #1=w895, index #2=w893, index #3=w901) -> (element #1=w907:string, element #2=w906:string, element #3=w900:string)
              n508 = Build Array(w902, w907, w905, w906, w905) -> (w904:string[])
              n509 = Decimal String To Number(string=w900) -> (number=w899:i32)  [unwired: 2 in, 1 out]
              n510 = Multiply(x=w899, y=12 ("x")) -> (x*y=w897:i32)
              n511 = Compound Arithmetic op=ADD(w897, 4, w895) -> (w894:i32)
            }
            n512 = Insert Into Array(array=string[][] [["", "", "", "", ""], ["", "", "", "", ""], ["", "", "", "", ""], ["", "", "", "", ""], ["", "", "", "", ""], ["", "", "", "", ""], ["", "", "", "", ""], ["", "", "", "", ""], ["", "", "", "", ""], ["", "", "", "", ""], ["", "", "", "", ""], ["", "", "", "", ""], ["", "", "", "", ""], ["", "", "", "", ""], ["", "", "", "", ""], ["", "", "", "", ""], ["", "", "", "", ""], ["", "", "", "", ""], ["", "", "", "", ""], ["", "", "", "", ""], ["", "", "", "", ""], ["", "", "", "", ""], ["", "", "", "", ""], ["", "", "", "", ""], ["", "", "", "", ""], ["", "", "", "", ""], ["", "", "", "", ""], ["", "", "", "", ""], ["", "", "", "", ""], ["", "", "", "", ""], ["", "", "", "", ""]], index (row)=0, new element=w882) -> (w881:string[][])  [unwired: 1 in]
            n513 = local write "Cycle Pattern"(w881) -> ()
          }
        }
      }
      frame "delete cycle" {
        n514 = Two Button Dialog(message="This operation will permanently delete this file!\nDo you want to continue?") -> (T button?=w917:bool)  [unwired: 2 in]
        n515 = case shown="True" w917 {
          tunnel: w916 -> [_ w922]
          frame False {
          }
          frame True {
            n516 = local read "Cycle List"() -> (w923:i32)
            n517 = property on="Cycle List" class="LstBox (strict)"() -> ("Item Names"=w924:string[])  [unwired: 2 in, 2 out]
            n518 = Index Array(array=w924, index=w923) -> (element=w921:string)
            n519 = Concatenate Strings(w922, w921) -> (w920:string)
            n520 = String To Path(string=w920) -> (path=w919:path)
            n521 = Delete(path (use dialog)=w919) -> ()  [unwired: 4 in, 3 out]
            n522 = local write "Flag 2"(FALSE) -> ()
          }
        }
      }
      frame "calc HC CO" {
        n523 = local read "Sub-Cycle Pattern"() -> (w941:string[][])
        n524 = Index Array(array=w941, index (col) #1=3 ("disabled index (col)"), index (col) #2=4 ("index (col)"), index (col) #3=11 ("index (col)")) -> (element #1=w931:string[], element #2=w938:string[], element #3=w925:string[])  [unwired: 3 in]
        n525 = Array Size(array=w931) -> (size(s)=w929:i32)
        n526 = Search 1D Array(1D array=w931, element="") -> (index of element=w928:i32)  [unwired: 1 in]
        n527 = Equal?(x=w928, y=-1) -> (x = y?=w930:bool)
        n528 = Select(t=w929, s=w930, f=w928) -> (s? t:f=w927:i32)
        n529 = for {
          N: w927 -> [_]
          tunnel: [w952] -> w935 mode=indexing
          tunnel: [w951] -> w934 mode=indexing
          tunnel: w931 -> [w950] mode=indexing
          tunnel: w938 -> [w949] mode=indexing
          tunnel: w925 -> [w948] mode=indexing
          w947 = ""
          n530 = Not Equal?(x=w950, y=w947) -> (x != y?=w946:bool)
          n531 = Not Equal?(x=w949, y=w947) -> (x != y?=w945:bool)
          n532 = Not Equal?(x=w948, y=w947) -> (x != y?=w944:bool)
          n533 = Compound Arithmetic op=AND(w946, w945, w944) -> (w943:bool)
          n534 = case shown="True" w943 {
            tunnel: w950 -> [_ w981]
            tunnel: w949 -> [_ w980]
            tunnel: [w953 w977] -> w951
            tunnel: [w953 w976] -> w952
            tunnel: w948 -> [_ w954]
            frame False {
              w953 = ""
            }
            frame True {
              # "O2Eq"
              n535 = Fract/Exp String To Number(string=w954) -> (number=w955:dbl)  [unwired: 3 in, 1 out]
              n536 = Fract/Exp String To Number(string=w981) -> (number=w962:dbl)  [unwired: 3 in, 1 out]
              n537 = Fract/Exp String To Number(string=w980) -> (number=w958:dbl)  [unwired: 3 in, 1 out]
              n538 = Decrement(x=w962) -> (x-1=w963:dbl)
              n539 = Divide(x=w955, y=20000.0) -> (x/y=w956:dbl)
              n540 = Multiply(x=4.76, y=w962) -> (x*y=w967:dbl)
              n541 = Multiply(x=w963, y=100.0) -> (x*y=w965:dbl)
              n542 = Add(x=w958, y=w956) -> (x+y=w959:dbl)
              n543 = Add(x=0.33, y=w967) -> (x+y=w969:dbl)
              n544 = Divide(x=w965, y=w969) -> (x/y=w970:dbl)
              n545 = Subtract(x=w959, y=w970) -> (x-y=w972:dbl)
              n546 = Multiply(x=w972, y=2.0) -> (x*y=w960:dbl)
              n547 = Divide(x=w972, y=5.0) -> (x/y=w961:dbl)
              n548 = Number To Fractional String(number=w961, width (-)=i16 6, precision (6)=i16 3) -> (F-format string=w976:string)  [unwired: 1 in]
              n549 = Number To Fractional String(number=w960, width (-)=i16 6, precision (6)=i16 2) -> (F-format string=w977:string)  [unwired: 1 in]
            }
          }
        }
        n550 = Replace Array Subset(array=w941, new element #1=w935, index (col) #1=5 ("disabled index (col)"), new element #2=w934, index (col) #2=6 ("disabled index (col)")) -> (w939:string[][])  [unwired: 2 in]
        n551 = local write "Sub-Cycle Pattern"(w939) -> ()
      }
      frame "Total time calc" {
        w996 = i16 2 ("width (-)")
        w1003 = ":"
        n552 = local read "Cycle Pattern"() -> (w1010:string[][])
        n553 = Index Array(array=w1010, index (col)=4 ("disabled index (col)")) -> (element=w983:string[])  [unwired: 1 in]
        n554 = Array Size(array=w983) -> (size(s)=w985:i32)
        n555 = Search 1D Array(1D array=w983, element="") -> (index of element=w984:i32)  [unwired: 1 in]
        n556 = Equal?(x=w984, y=-1) -> (x = y?=w986:bool)
        n557 = Select(t=w985, s=w986, f=w984) -> (s? t:f=w982:i32)
        n558 = for {
          N: w982 -> [_]
          tunnel: w983 -> [w1018] mode=indexing
          shift-right: [w1020] -> w1006
          shift-left: 0 -> [w1021]
          n559 = xnode "Match Regular Expression"("input string"=w1018, "regular expression"=":" ("search string/char (-)")) -> ("before match"=w1017:string, "after match"=w1014:string)  [unwired: 4 in, 3 out]
          n560 = Decimal String To Number(string=w1017) -> (number=w1016:i32)  [unwired: 2 in, 1 out]
          n561 = Decimal String To Number(string=w1014) -> (number=w1013:i32)  [unwired: 2 in, 1 out]
          n562 = Multiply(x=w1016, y=60) -> (x*y=w1012:i32)
          n563 = Add(x=w1012, y=w1013) -> (x+y=w1011:i32)
          n564 = Add(x=w1011, y=w1021) -> (x+y=w1020:i32)
        }
        n565 = local read "Total Number of Cycles"() -> (w1007:T1)
        n566 = Multiply(x=w1006, y=w1007) -> (x*y=w1002:T1)
        n567 = Quotient & Remainder(x=w1002, y=3600.0) -> (x-y*floor(x/y)=w989:T1, floor(x/y)=w999:T1)
        n568 = Quotient & Remainder(x=w989, y=60.0) -> (x-y*floor(x/y)=w997:T1, floor(x/y)=w998:T1)
        n569 = Number To Decimal String(number=w999) -> (decimal integer string=w1004:string)  [unwired: 1 in]
        n570 = Number To Decimal String(number=w998, width (-)=w996) -> (decimal integer string=w1000:string)
        n571 = Number To Decimal String(number=w997, width (-)=w996) -> (decimal integer string=w995:string)
        n572 = Concatenate Strings(w1004, w1003, w1000, w1003, w995) -> (w994:string)
        n573 = call <vilib>:"Search and Replace Pattern.vi"("string"=w994, "regular expression (\"\")"=" " ("replace string (\"\")"), "replace string (\"\")"="0" ("replace string (\"\")"), "replace all? (F)"=TRUE) -> ("result string"=→"Total Test Duration (hrs)":string)  [unwired: 1 in, 1 out]
      }
      frame "update Cycle pattern " {
        n574 = local read "Cycle Pattern"() -> (w1149:string[][])
        n575 = Index Array(array=w1149, index (col)=1 ("disabled index (col)")) -> (element=w1134:string[])  [unwired: 1 in]
        n576 = String To Path(string=w1151) -> (path=w1152:path)
        n577 = Array Size(array=w1134) -> (size(s)=w1137:i32)
        n578 = Search 1D Array(1D array=w1134, element="") -> (index of element=w1136:i32)  [unwired: 1 in]
        n579 = List Folder(path=w1152, pattern="*.eyes") -> (filenames=w1150:string[])  [unwired: 2 in, 3 out]
        n580 = Equal?(x=w1136, y=-1) -> (x = y?=w1138:bool)
        n581 = Select(t=w1137, s=w1138, f=w1136) -> (s? t:f=w1135:i32)
        n582 = for {
          N: w1135 -> [_]
          tunnel: w1149 -> [w1168] mode=indexing
          tunnel: w1151 -> [w1161]
          tunnel: [w1163] -> w1144 mode=indexing
          tunnel: [w1165] -> w1148 mode=indexing
          tunnel: [w1162] -> w1145 mode=indexing
          tunnel: w1150 -> [w1160]
          tunnel: [w1155] -> w1141 mode=indexing
          n583 = Index Array(array=w1168, index #1=1 ("index"), index #2=3 ("index")) -> (element #1=w1159:string, element #2=w1164:string)
          n584 = Search 1D Array(1D array=w1160, element=w1159) -> (index of element=w1158:i32)  [unwired: 1 in]
          n585 = Not Equal?(x=w1158, y=-1) -> (x != y?=w1156:bool)
          n586 = case shown="True" w1156 {
            tunnel: [w1172 w1186] -> w1165
            tunnel: w1164 -> [_ w1182]
            tunnel: [w1172 w1180] -> w1163
            tunnel: [w1172 w1179] -> w1162
            tunnel: w1161 -> [_ w1178]
            tunnel: w1159 -> [w1171 w1177]
            tunnel: [w1170 w1177] -> w1155
            frame False {
              w1172 = "N/A" ("String")
              n587 = Concatenate Strings(w1171, " - File NOT AVAILABLE !!!" ("string")) -> (w1170:string)
            }
            frame True {
              w1190 = i16 2 ("width (-)")
              n588 = Concatenate Strings(w1178, w1177) -> (w1208:string)
              n589 = String To Path(string=w1208) -> (path=w1207:path)
              n590 = call <vilib>:"Search and Replace Pattern.vi"("string"=w1182, "regular expression (\"\")"="[a-x ]" ("format string"), "replace string (\"\")"="", "replace all? (F)"=TRUE) -> ("result string"=w1179:string)  [unwired: 1 in, 1 out]
              n591 = call-poly <vilib>:"Read From Spreadsheet File.vi"("file path (dialog if empty)"=w1207) -> ("first row"=w1176:string[])  [unwired: 6 in, 4 out]
              n592 = Delete From Array(array=w1176, length=1, index=0) -> (array with subset deleted=w1175:string[])  [unwired: 1 out]
              n593 = Array Size(array=w1175) -> (size(s)=w1206:i32)
              n594 = Equal?(x=w1179, y="") -> (x = y?=w1194:bool)
              n595 = Subtract(x=w1206, y=12) -> (x-y=w1204:i32)
              n596 = Select(t="0", s=w1194, f=w1179) -> (s? t:f=w1193:string)
              n597 = Index Array(array=w1175, index=w1204) -> (element=w1180:string)
              n598 = Decimal String To Number(string=w1193) -> (number=w1203:i32)  [unwired: 2 in, 1 out]
              n599 = Decimal String To Number(string=w1180) -> (number=w1202:i32)  [unwired: 2 in, 1 out]
              n600 = Multiply(x=w1203, y=w1202) -> (x*y=w1201:i32)
              n601 = Quotient & Remainder(x=w1201, y=60) -> (x-y*floor(x/y)=w1199:i32, floor(x/y)=w1198:i32)
              n602 = Number To Decimal String(number=w1199, width (-)=w1190) -> (decimal integer string=w1196:string)
              n603 = Number To Decimal String(number=w1198, width (-)=w1190) -> (decimal integer string=w1195:string)
              n604 = Concatenate Strings(w1195, ":", w1196) -> (w1189:string)
              n605 = call <vilib>:"Search and Replace Pattern.vi"("string"=w1189, "regular expression (\"\")"=" " ("replace string (\"\")"), "replace string (\"\")"="0" ("replace string (\"\")"), "replace all? (F)"=TRUE) -> ("result string"=w1186:string)  [unwired: 1 in, 1 out]
            }
          }
        }
        n606 = Replace Array Subset(array=w1149, new element #1=w1141, index (col) #1=1 ("disabled index (col)"), new element #2=w1144, index (col) #2=2 ("disabled index (col)"), new element #3=w1145, index (col) #3=3 ("disabled index (col)"), new element #4=w1148, index (col) #4=4 ("disabled index (col)")) -> (w1153:string[][])  [unwired: 4 in]
        n607 = local write "Cycle Pattern"(w1153) -> ()
      }
      frame "load cycle name" {
        n608 = property on="Cycle Pattern" class="Tbl (strict)"() -> ("EditPos"=w1214:T3)  [unwired: 2 in, 2 out]
        n609 = Unbundle By Name(w1214) -> ("Row"=w1212:i32, "Column"=w1211:i32)
        n610 = local read "Cycle Pattern"() -> (w1210:string[][])
        n611 = call "SubCycles list.vi"() -> ("Subcycle name"=w1213:string)  [unwired: 10 in, 1 out]
        n612 = Replace Array Subset(array=w1210, new element=w1213, index (row)=w1212, index (col)=w1211) -> (w1209:string[][])
        n613 = local write "Cycle Pattern"(w1209) -> ()
      }
      frame "load test array" {
        n614 = local read "Total Test Duration (hrs)"() -> (w1222:T8)
        n615 = local read "Cycle Name"() -> (w1218:T5)
        n616 = Equal?(x=w1218, y="") -> (x = y?=w1217:bool)
        n617 = Not Equal?(x=w1222, y="0:00:00") -> (x != y?=w1216:bool)
        n618 = Or(x=w1216, y=w1217) -> (x .or. y?=w1215:bool)
        n619 = case shown="True" w1215 {
          selector: w1215 -> [w1223 _]
          tunnel: [FALSE TRUE] -> w1220
          frame False {
            n620 = case shown="False" w1223 {
              frame False {
                n621 = One Button Dialog(message="Incomplete Data!\nReview the cycle pattern!") -> ()  [unwired: 1 in, 1 out]
              }
              frame True {
              }
            }
          }
          frame True {
            w1229 = 0.0 ("default (0 I32)")
            n622 = local read "Cycle Name"() -> (w1244:T5)
            n623 = Concatenate Strings("C:\\Setup Files\\Cycles Folder\\", w1244, ".eyec" ("string")) -> (w1242:string)
            n624 = String To Path(string=w1242) -> (path=w1243:path)
            n625 = local read "Total Number of Cycles"() -> (w1240:T1)
            n626 = call-poly <vilib>:"Read From Spreadsheet File.vi"("file path (dialog if empty)"=w1243) -> ("first row"=w1226:string[])  [unwired: 6 in, 4 out]
            n627 = call "Remove names.vi"("Array in"=w1226) -> ("Array out"=w1235:string[])  [unwired: 10 in]
            n628 = Index Array(array=w1226, index #1=14 ("index"), index #2=15 ("index")) -> (element #1=w1231:string, element #2=w1227:string)
            n629 = Number To Decimal String(number="Ageing Gas") -> (decimal integer string=w1239:string)  [unwired: 1 in]
            n630 = Number To Decimal String(number=w1240) -> (decimal integer string=w1238:string)  [unwired: 1 in]
            n631 = Decimal String To Number(string=w1227, default (0L)=w1229) -> (number=w1228:dbl)  [unwired: 1 in, 1 out]
            n632 = Decimal String To Number(string=w1231, default (0L)=w1229) -> (number=w1230:dbl)  [unwired: 1 in, 1 out]
            n633 = property on="Inlet temp Age" class="DigNum (strict)"("Value"=w1230) -> ()  [unwired: 2 in, 2 out]
            n634 = property on="Flow rate Age" class="DigNum (strict)"("Value"=w1228) -> ()  [unwired: 2 in, 2 out]
            n635 = Build Array (concatenate)(w1239, w1238, w1235) -> (w1234:string[])
            n636 = shared-variable "cRIO-9082\\Library 1.lvlib\\Ageing Variables"(w1234) -> ()  [unwired: 1 in, 1 out]
          }
        }
        "Test Compiled" <- w1220
      }
      frame "convert to num" {
        n637 = local read "EditPos Subc"() -> (w1249:T3)
        n638 = Unbundle By Name(w1249) -> ("Row"=w1250:i32, "Column"=w1247:i32)
        n639 = Equal?(x=w1247, y=7) -> (x = y?=w1246:bool)
        n640 = case shown="False" w1246 {
          tunnel: w1250 -> [_ w1255]
          tunnel: w1247 -> [_ w1253]
          tunnel: w1249 -> [_ _]
          frame True {
          }
          frame False {
            n641 = local read "Sub-Cycle Pattern"() -> (w1252:string[][])
            n642 = call "Conv to num.vi"("Column"=w1253, "Row"=w1255, "Array"=w1252) -> ("result string"=w1254:string)  [unwired: 8 in]
            n643 = Replace Array Subset(array=w1252, new element=w1254, index (row)=w1255, index (col)=w1253) -> (w1251:string[][])
            n644 = local write "Sub-Cycle Pattern"(w1251) -> ()
          }
        }
      }
      frame "check scycle name" {
        n645 = local read "Sub-Cycle Name"() -> (w1256:T5)
        n646 = call <vilib>:"Search and Replace Pattern.vi"("string"=w1256, "regular expression (\"\")"="[^0-9a-zA-Z ]" ("format string"), "replace string (\"\")"="", "replace all? (F)"=TRUE) -> ("result string"=w1262:string)  [unwired: 1 in, 1 out]
        n647 = Not Equal?(x=w1262, y=w1256) -> (x != y?=w1261:bool)
        n648 = case shown="False" w1261 {
          tunnel: w1262 -> [w1263 w1264]
          tunnel: [w1263 w1264] -> w1257
          frame False {
          }
          frame True {
            n649 = One Button Dialog(message="Unsuitable character for the file name!") -> ()  [unwired: 1 in, 1 out]
          }
        }
        n650 = local write "Sub-Cycle Name"(w1257) -> ()
      }
      frame "check cycle name" {
        n651 = local read "Cycle Name"() -> (w1266:T5)
        n652 = call <vilib>:"Search and Replace Pattern.vi"("string"=w1266, "regular expression (\"\")"="[^0-9a-zA-Z ]" ("format string"), "replace string (\"\")"="", "replace all? (F)"=TRUE) -> ("result string"=w1272:string)  [unwired: 1 in, 1 out]
        n653 = Not Equal?(x=w1272, y=w1266) -> (x != y?=w1271:bool)
        n654 = case shown="False" w1271 {
          tunnel: w1272 -> [w1273 w1274]
          tunnel: [w1273 w1274] -> w1267
          frame False {
          }
          frame True {
            n655 = One Button Dialog(message="Unsuitable character for the file name!") -> ()  [unwired: 1 in, 1 out]
          }
        }
        n656 = local write "Cycle Name"(w1267) -> ()
      }
      frame "Multigas connect" {
        # "add here logic to verify the user requirements and the machine state\n0 - not connected\n1 - MKS1 & Ext An Up\n2 - MKS2 & Ext An Dn\n3 - MKS 1 & 2  & Ext An Up & Dn"
        n657 = flat-sequence {
          frame #0 {
            "Connected?" <- TRUE
          }
        }
      }
      frame "Multigas disconnect" {
      }
    }
    n658 = local read "stop 2"() -> (w656:bool)
  }
  n659 = node-c288(w1) -> ()  [unwired: 1 out]
  n660 = local write "stop 2"(w11) -> ()
  n661 = disable-structure shown="Disabled" {
    frame Disabled {
      n662 = while {
        tunnel: [w1315] -> w1300
        tunnel: [w1314] -> w1299
        stop <- w1311 stop-if-true
        n663 = TCP Open Connection(address="192.168.1.3", remote port or service name=u16 7700) -> (connection ID=w1315:refnum<k5>, error out=w1314:errorcluster)  [unwired: 3 in]
        n664 = Unbundle By Name(w1314) -> ("status"=w1316:bool)
        n665 = Not(x=w1316) -> (.not. x?=w1312:bool)
        n666 = Or(x=w1312, y="stop TCP") -> (x .or. y?=w1311:bool)
      }
      n667 = Concatenate Strings("\r", "\n") -> (w1288:string)
      n668 = Concatenate Strings("MSSM,0,1,1" ("data in"), w1288) -> (w1295:string)
      n669 = TCP Write(connection ID=w1300, data in=w1295, error in (no error)=w1299) -> (connection ID out=w1303:refnum<k5>, error out=w1304:errorcluster)  [unwired: 1 in, 1 out]
      n670 = Concatenate Strings("MSMD,1,7,1,1,1,1,2,1,1,3,1,1,4,1,1,5,1,1,6,1,1,7,1" ("data in"), w1288) -> (w1290:string)
      n671 = TCP Write(connection ID=w1303, data in=w1290, error in (no error)=w1304) -> (connection ID out=w1301:refnum<k5>, error out=w1302:errorcluster)  [unwired: 1 in, 1 out]
      n672 = Concatenate Strings("MSTT,1,0" ("string"), w1288) -> (w1289:string)
      n673 = TCP Write(connection ID=w1301, data in=w1289, error in (no error)=w1302) -> (connection ID out=w1287:refnum<k5>, error out=w1286:errorcluster)  [unwired: 1 in, 1 out]
      n674 = UDP Open(9:500 ("timeout ms (25000)"), 11:u16 7701 ("port")) -> ()  [unwired: 3 in, 3 out]
      n675 = UDP Read(timeout ms (25000)=500) -> (data out=w1278:string)  [unwired: 3 in, 4 out]
      n676 = while {
        shift-right: [w1307] -> _
        shift-left: w1278 -> [w1310]
        tunnel: [w1308] -> w1279 mode=indexing
        stop <- w1305 stop-if-true
        n677 = Search/Split String(string=w1310, search string/char (-)=",") -> (substring before match=w1308:string, match + rest of string=w1307:string)  [unwired: 1 in, 1 out]
        n678 = String Length(string=w1307) -> (length=w1306:i32)
        n679 = Equal To 0?(x=w1306) -> (x = 0?=w1305:bool)
      }
      n680 = call "7170string to array.vi"("Array in"=w1279) -> ()  [unwired: 4 in, 1 out]
      n681 = UDP Close() -> ()  [unwired: 2 in, 2 out]
      n682 = Concatenate Strings("MSTP,0,0" ("string"), "\r", "\n") -> (w1282:string)
      n683 = TCP Write(data in=w1282) -> (connection ID out=w1284:refnum<k5>, error out=w1285:errorcluster)  [unwired: 3 in, 1 out]
      n684 = TCP Close Connection(connection ID=w1284, error in (no error)=w1285) -> ()  [unwired: 1 in, 2 out]
    }
    frame Enabled {
    }
  }
  n685 = node-c288(w8) -> ()  [unwired: 1 out]
  "Table" <- string[][] [] ("Table")
